vi "VP_RT_dual.vi"() -> ()   [LabVIEW 2015]
uses:
  State Enum.ctl
  Command Enum.ctl
  Controller Type.ctl
  Scan type.ctl
  EPICS Command Control.ctl
  <vilib>/Platform/TimedLoop/XDataNode/timing_clust.ctl
  <vilib>/Platform/TimedLoop/XDataNode/nitl_modes.ctl
  <vilib>/Platform/TimedLoop/XDataNode/wakeup.ctl
  Data Write Control.ctl
  <vilib>/FPGAPlugInAG/cRIO-9039/niLvFpga_Open_cRIO-9039.vi
  <vilib>/rvi/interface/common/dynamic/niFpgaDynamicAddResources.vi
  <vilib>/Utility/error.llb/Error Cluster From Error Code.vi
  <vilib>/rvi/errors/niLvFpgaAdjustHostInterfaceError.vi
  <vilib>/rvi/interface/common/niFpgaWaitOnOcc.vi
  <vilib>/FPGAPlugInAG/Dynamic/niLvFpga_Reset_Dynamic.vi
  <vilib>/FPGAPlugInAG/Dynamic/niLvFpga_Abort_Dynamic.vi
  <vilib>/FPGAPlugInAG/Dynamic/niLvFpga_Close_Dynamic.vi
  <vilib>/Platform/TimedLoop/XDataNode/XDataNode.xnode
  <vilib>/rvi/interface/nirviOpenFPGA/nirviOpenFPGA.xnode
  FPGA Bitfiles/VP_NanoPositioner_FPGA_Diagonal.lvbitx
  <vilib>/rvi/interface/nirviReadWriteControl/nirviReadWriteControl.xnode
  <vilib>/rvi/interface/nirviMethod/nirviMethod.xnode
  <vilib>/rvi/interface/nirviCloseFPGA/nirviCloseFPGA.xnode
  <vilib>/Platform/TimedLoop/XDataNode/XDNodeRunTimeDep.lvlib
  <vilib>/rvi/errors/niLvFpgaMergeErrorWithErrorCode.vi
  NiFpgaLv.dll
  <vilib>/rvi/interface/Simulation/niFpgaSimulationCallBeginRW.vi
  <vilib>/rvi/Analysis/host/Public/NI_FpgaMspHost.lvlib
  <vilib>/FPGAPlugInAG/Dynamic/niLvFpga_StopFifo_Dynamic.vi
  <vilib>/FPGAPlugInAG/Dynamic/niLvFpga_ReadFifo_Dynamic.vi
  <vilib>/NI_Real-Time Target Support.lvlib
  <vilib>/FPGAPlugInAG/Dynamic/niLvFpga_ConfigureFifo_Dynamic.vi
panel:
  in  "Tab Control":T1(tab)
  in  "Scan type":T2
  in  "Controller Type":T3
  out "Fly Scan Complete":bool
  out "XY actual":cluster{"Array":dbl[], "Array":dbl[]}(graph)
  out "XY Ref":cluster{"Array":dbl[], "Array":dbl[]}(graph)
  out "Elements Available in FIFO":u32(graph)
  out "Elements Remaining in FIFO":u32(graph)
  out "Reference and Actual positions":cluster{"t0":dbl, dbl, dbl[][]}(graph)
  in  "Timeout FPGA FIFO1":i32=40000000
  out "FIFO Timed Out":bool
  out "stop case":bool
  in  "Datalog Cases":T4(ring)=enum."Data Log 16"
  out "FIFO Timed Out?":bool
  in  "FIFO Time Period":dbl=0.01 format="%#_13g"
  out "Number of Elements":u32=1250
  out "Datalog Rate (Hz)":dbl=25000.000000000004
  out "Elements Remaining":u32
  in  "Timeout (ms)":i32=10000
  out "Actual Depth":u32=131068416
  in  "Requested Depth":u32=131068000
  out "2iddVELO:VP:X_End_nm":dbl=2000.0
  out "2iddVELO:VP:X_Start_nm":dbl=-2000.0
  out "EPICS Execute Command":bool
  out "2iddVELO:VP:Y_Start_nm":dbl=2000.0
  out "2iddVELO:VP:Y_End_nm":dbl=-2000.0
  out "2iddVELO:VP:Y_Step_Size_nm":dbl=50.0
  out "2iddVELO:VP:X_Step_Size_nm":dbl=50.0
  out "2iddVELO:VP:Trigger_Freq_Hz":dbl=1000.0
  out "2iddVELO:VP:Trig_DutyCycle_Per":dbl=99.0
  out "Iteration Duration RT Timed-Loop":i64=128
  in  "X Ramp Start (nm)":fxp<+/-,16,16>=-500.0
  in  "X Ramp End (nm)":fxp<+/-,16,16>=500.0
  in  "X Start Marker (nm)":fxp<+/-,58,25>
  in  "Y Ramp Start (nm)":fxp<+/-,16,16>=500.0
  in  "Y Ramp End (nm)":fxp<+/-,16,16>=-500.0
  in  "Y Step Size (nm)":fxp<+/-,16,16>=50.0
  in  "Y Start Marker (nm)":fxp<+/-,58,25>
  out "Fly Scan Running":bool
  out "Continue Run":bool
  out "X Ramp Period (usec)":fxp<+,24,24>=60000.0
  out "Y Ramp Period (usec)":fxp<+,24,24>=60000.0
  out "# of Hor Lines":fxp<+/-,34,18>=181.0 format="%.22g"
  in  "X Step Size (nm)":fxp<+/-,16,16>=50.0
  out "# of Points per Line":fxp<+/-,33,17>=180.0
  out "# Total Trigger Points":fxp<+/-,64,34>=32580.0
  out "sec per line":dbl=0.06
  out "line per sec (Hz)":dbl=16.666666666666668
  out "X Ramp Period DBL (usec)":dbl=60000.0 format="%#_6f"
  out "Total Scan Time (sec)":dbl=10.86
  in  "Controller Time Period (uSec)":u32=40
  in  "Controller Output Time Period (uSec)":u32=40
  in  "X Reference Time Period (uSec)":u32=40
  in  "Plant Output Time Period (uSec)":u32=40
  in  "Stop System (Careful!!)":bool
  in  "Datalog Time Period (uSec)":u32=40
  in  "Analog Input Time Period (uSec)":u32=40
  in  "Detector Trigger Time Period (uSec)":u32=40
  in  "Trigger Generation Time Period (uSec)":u32=40
  in  "Y Reference Time Period (uSec)":u32=40
  in  "Z Reference Time Period (uSec)":u32=40
  in  "Data Trigger Time Period (uSec)":u32=40
  in  "Reset All":bool
  in  "System Loop Type":enum16{"Open Loop", "Closed Loop"}(ring)
  in  "Base name":string="base_name"
  out "Trigger for Data":fxp<+/-,58,25>=1.0
  out "Data":fxp<+/-,58,25>[](array[numeric])
  out "Number of Data Strings":i32=5
  out "Mod6/DIO3":bool
  out "Mod5/DIO3":bool
  out "Mod4/DIO3":bool
  in  "Sample Z Stage Resolution (nm)":fxp<+,33,3>=0.5
  in  "Sample Y Stage Resolution (nm)":fxp<+,33,3>=0.5
  in  "Sample X Stage Resolution (nm)":fxp<+,33,3>=0.5
  in  "Optics Z Stage Resolution (nm)":fxp<+,33,3>=0.5
  in  "Optics Y Stage Resolution (nm)":fxp<+,33,3>=0.5
  in  "Optics X Stage Resolution (nm)":fxp<+,33,3>=0.5
  in  "Sample Z Reset":bool
  in  "Sample Y Reset":bool
  in  "Sample X Reset":bool
  out "Mod6/DIO2":bool
  out "Mod6/DIO1":bool
  out "Mod6/DIO0":bool=TRUE
  out "Mod5/DIO2":bool
  out "Mod5/DIO1":bool=TRUE
  out "Mod5/DIO0":bool
  out "Mod4/DIO2":bool=TRUE
  out "Mod4/DIO1":bool
  out "Mod4/DIO0":bool=TRUE
  in  "Optics Z Reset":bool
  in  "Optics Y Reset":bool
  in  "Optics X Reset":bool
  in  "Detector Trigger Lower Limit (V)":fxp<+/-,20,5>
  in  "Detector Trigger Upper Limit (V)":fxp<+/-,20,5>=5.0
  out "Detector Trigger (V)":fxp<+/-,20,5>
  out "Detector Trigger In Range?":bool=TRUE
  in  "Trigger High Period (usec)":fxp<+/-,64,45>=1250.0
  in  "Trigger Low Period (usec)":fxp<+/-,64,45>=1250.0
  in  "Trigger High Level (V)":fxp<+/-,20,5>=5.0
  in  "Trigger Low Level (V)":fxp<+/-,20,5>
  in  "Trigger Wave Generator":T5(ring)=enum."Square Wave 1"
  in  "DT Reference Amplitude (V)":fxp<+/-,40,17>=5.0
  in  "DT Reference DC Offset (V)":fxp<+/-,16,16>
  out "DT Frequency (periods/tick)":fxp<+,32,0>=7.500010542571545e-05
  out "DT Phase Offset (periods)":fxp<+,32,0>
  in  "DT Reset":bool
  out "DT Duty Cycle (periods)":fxp<+,32,0>=0.8799999998882413
  in  "DT phase offset (deg)":dbl format="%#.6g"
  in  "DT Frequency (Hz)":dbl=200.0 format="%#_6p"
  in  "DT duty cycle (%)":dbl=88.0 min=0.0 max=100.0 step=1.0
  in  "Z White Noise Seed":u32=4
  in  "Z White Noise Amplitude":u16=32767
  in  "Y White Noise Seed":u32=4
  in  "Y White Noise Amplitude":u16=32767
  in  "Z Reference Reset":bool
  in  "Y Reference Reset":bool
  in  "X Reference Reset":bool
  in  "Z Reference Wave Selection":T6(ring)=enum."Sine Wave"
  in  "X Reference Wave Selection":T7(ring)=enum."Custom Up Down Ramp"
  in  "Y Reference Wave Selection":T8(ring)=enum."Custom Ramp Wave"
  out "Z phase offset (periods)":fxp<+,32,0>
  out "Z frequency (periods/tick)":fxp<+,32,0>=1.25030055642128e-07 format="%.32g"
  in  "Z phase offset (deg)":dbl format="%#.6g"
  in  "Z frequency (Hz)":dbl=5.0 format="%#_6p"
  out "Y phase offset (periods)":fxp<+,32,0>
  out "Y frequency (periods/tick)":fxp<+,32,0>=5.005858838558197e-08 format="%.32g"
  in  "Y phase offset (deg)":dbl format="%#.6g"
  in  "Y frequency (Hz)":dbl=2.0 format="%#_6p"
  out "Z Stage Reference (nm)":fxp<+/-,58,25>
  out "Y Stage Reference (nm)":fxp<+/-,58,25>
  out "X Stage Reference (nm)":fxp<+/-,58,25>
  in  "X White Noise Seed":u32=4
  in  "X White Noise Amplitude":u16=32767
  in  "Z Reference DC Offset (nm)":fxp<+/-,15,15>
  in  "Y Reference DC Offset (nm)":fxp<+/-,16,16>
  in  "X Reference DC Offset (nm)":fxp<+/-,16,16>
  in  "Z Reference Amplitude (nm)":fxp<+/-,40,17>
  in  "Y Reference Amplitude (nm)":fxp<+/-,40,17>=100.0
  in  "X Reference Amplitude (nm)":fxp<+/-,40,17>=100.0
  out "X phase offset (periods)":fxp<+,32,0>
  out "X frequency (periods/tick)":fxp<+,32,0>=1.25030055642128e-07 format="%.32g"
  in  "X phase offset (deg)":dbl format="%#.6g"
  in  "X frequency (Hz)":dbl=5.0 format="%#_6p"
  in  "Scaling mV to V":fxp<+,33,10>=0.001000046730041504
  out "Heartbeat":bool=TRUE
  in  "System command":T9
  in  "Execute":bool
  out "Last Command Executed":T9
  in  "Optics and or Sample Stage":T10(ring)
  out "Remote Mode":bool
  in  "Local_Lock":bool
  out "Snake Scan Reference FPGA or EPICS":enum16{"FPGA Snake Scan", "EPICS Snake Scan"}(ring)
  out "Output filename":string
  out "Output path":path
  out "FPGA state":T11(ring)
  in  "cRIO data dir":string="/home/lvuser/natinst/data"
  out "RT Main Loop State":T12
  out "cRIO path":path
  out "Trigger Frequency (Hz)":dbl
  out "Trigger Duty Cycle (%)":dbl
  out "EPICS Scan Type":T2
  out "EPICS Controller Type":T3
  out "EPICS cRIO Command":T13
  out "Scan loop dt":i64
  in  "Z-Stage Scaling Direction":fxp<+/-,3,3>=-1.0
  in  "Y-Stage Scaling Direction":fxp<+/-,3,3>=-1.0
  in  "Mod 3 AI2 V to nm Scaling":fxp<+,47,18>=1000.0
  in  "Mod 3 AI1 V to nm Scaling":fxp<+,47,18>=1000.0
  in  "Mod 3 AI0 V to nm Scaling":fxp<+,47,18>=1000.0
  out "PI Z-Stage Input (V)":fxp<+/-,20,5>=-0.000732421875
  out "PI Y-Stage Input (V)":fxp<+/-,20,5>=0.005584716796875
  out "PI X-Stage Input (V)":fxp<+/-,20,5>=-0.00311279296875
  in  "Z-Stage nm to V Scaling":fxp<+/-,32,12>=0.0005397796630859375
  in  "Y-Stage nm to V Scaling":fxp<+/-,32,12>=0.0014200210571289062
  in  "X-Stage Scaling Direction":fxp<+/-,3,3>=-1.0
  in  "X-Stage nm to V Scaling":fxp<+/-,32,12>=0.0005359649658203125
  in  "Controller Output Lower Limit":fxp<+/-,20,5>=-5.0
  in  "Controller Output Upper Limit":fxp<+/-,20,5>=5.0
  in  "FPGA Wait Timer (ms)":u16=50
  in  "Pre-Scan pause (ms)":u32=250
  in  "Readback Loop time between iterations (ms)":u32=10
  out "Measured Datalog Time Period (Ticks)":u32=1600
  out "Measured Datalog Loop Rate (secs)":dbl=3.9999999999999996e-05
  out "Measured Datalog Loop Rate (kHz)":dbl=25.000000000000004
  out "Measured Counter Loop Rate (secs)":dbl
  out "Measured Counter Loop Rate (MHz)":dbl=inf
  out "Measured X Reference Loop Rate (secs)":dbl=3.9999999999999996e-05
  out "Measured X Reference Loop Rate (kHz)":dbl=25.000000000000004
  out "Measured X Reference Time Period (Ticks)":u32=1600
  out "Measured Controller Loop Rate (kHz)":dbl=25.000000000000004
  out "Measured Controller Output Loop Rate (secs)":dbl=3.9999999999999996e-05
  out "Measured Controller Output Loop Rate (kHz)":dbl=25.000000000000004
  out "Measured Plant Output Loop Rate (secs)":dbl=3.9999999999999996e-05
  out "Measured Plant Output Loop Rate (kHz)":dbl=25.000000000000004
  out "Measured Controller Loop Rate (secs)":dbl=3.9999999999999996e-05
  out "Measured Controller Time Period (Ticks)":u32=1600
  out "Datalog Time Period (sec)":dbl=3.9999999999999996e-05
  out "Measured Controller Output Time Period (Ticks)":u32=1600
  out "Measured Plant Output Time Period (Ticks)":u32=1600
  out "Measured Counter Time Period (Ticks)":u32
  out "32 bit Count Optics X":i32
  out "32 bit Count Optics  Y":i32
  out "32 bit Count Optics  Z":i32
  out "32 bit Count Sample X":i32
  out "32 bit Count Sample  Y":i32=2
  out "32 bit Count Sample  Z":i32=-4
  out "Optics X Stage Displacement (nm)":fxp<+/-,58,25>=-1.0
  out "Optics Y Stage Displacement (nm)":fxp<+/-,58,25>
  out "Optics Z Stage Displacement (nm)":fxp<+/-,58,25>
  out "Sample X Stage Displacement (nm)":fxp<+/-,58,25>=-0.5
  out "Sample Y Stage Displacement (nm)":fxp<+/-,58,25>=1.5
  out "Sample Z Stage Displacement (nm)":fxp<+/-,58,25>=-1.0
  out "Measured Analog Input Time Period (Ticks)":u32=1600
  out "Measured Analog Input Loop Rate (secs)":dbl=3.9999999999999996e-05
  out "Measured Analog Input Loop Rate (kHz)":dbl=25.000000000000004
  out "Measured Detector Trigger Time Period (Ticks)":u32=1600
  out "Measured Trigger Gen Time Period (Ticks)":u32=1600
  out "Measured Y Reference Time Period (Ticks)":u32=1600
  out "Measured Z Reference Time Period (Ticks)":u32=1600
  out "Measured Y Reference Loop Rate (secs)":dbl=3.9999999999999996e-05
  out "Measured Y Reference Loop Rate (kHz)":dbl=25.000000000000004
  out "Measured Z Reference Loop Rate (secs)":dbl=3.9999999999999996e-05
  out "Measured Z Reference Loop Rate (kHz)":dbl=25.000000000000004
  out "Measured Data Trigger Time Period (Ticks)":u32=1600
  out "X-Stage Input In Range?":bool=TRUE
  out "Y-Stage Input In Range?":bool=TRUE
  out "Z-Stage Input In Range?":bool=TRUE
  in  "file path soscoeff_xx1 Hinf":path=path "/home/lvuser/natinst/controllers/Kxx_1_Gxx_matched_dow_16ord_mVpnm_cd8a3_AvTio9_X5nm_500pm_all_40us_soscof_xx1.mat"
  in  "file path sos gain SF Controller_xx1 Hinf":path=path "/home/lvuser/natinst/controllers/Kxx_1_Gxx_matched_dow_16ord_mVpnm_cd8a3_AvTio9_X5nm_500pm_all_40us_soscof_xx2.mat"
  in  "file path soscoeff_yy1 Hinf":path=path "/home/lvuser/natinst/controllers/Kyy_trial_1_Gyy_matched_dow_8ord_mVpnm_cd8a3_AvTio9_Y5nm_500pm_all_40us_soscof_yy1.mat"
  in  "file path sos gain SF Controller_yy1 Hinf":path=path "/home/lvuser/natinst/controllers/Kyy_trial_1_Gyy_matched_dow_8ord_mVpnm_cd8a3_AvTio9_Y5nm_500pm_all_40us_soscof_yy2.mat"
  in  "file path soscoeff_zz1 Hinf":path=path "/home/lvuser/natinst/controllers/Kzz_1_Gzz_matched_dow_29ord_mVpnm_cd8a3_AvTio9_Z5nm_500pm_all_40us_soscof_zz1.mat"
  in  "file path sos gain SF Controller_zz1 Hinf":path=path "/home/lvuser/natinst/controllers/Kzz_1_Gzz_matched_dow_29ord_mVpnm_cd8a3_AvTio9_Z5nm_500pm_all_40us_soscof_zz2.mat"
  in  "file path soscoeff_xx1 PID":path=path "/home/lvuser/natinst/controllers/Kxx_pid_2_Gxx_tustin_2ord_mVpnm_cd8a3_soscof_xx1.mat"
  in  "file path sos gain SF Controller_xx1 PID":path=path "/home/lvuser/natinst/controllers/Kxx_pid_2_Gxx_tustin_2ord_mVpnm_cd8a3_soscof_xx2.mat"
  in  "file path soscoeff_yy1 PID":path=path "/home/lvuser/natinst/controllers/Kyy_pid_4_Gyy_tustin_2ord_mVpnm_cd8a3_soscof_yy1.mat"
  in  "file path sos gain SF Controller_yy1 PID":path=path "/home/lvuser/natinst/controllers/Kyy_pid_4_Gyy_tustin_2ord_mVpnm_cd8a3_soscof_yy2.mat"
  in  "file path soscoeff_zz1 PID":path=path "/home/lvuser/natinst/controllers/Kzz_pid_2_Gzz_tustin_2ord_mVpnm_cd8a3_soscof_zz1.mat"
  in  "file path sos gain SF Controller_zz1 PID":path=path "/home/lvuser/natinst/controllers/Kzz_pid_2_Gzz_tustin_2ord_mVpnm_cd8a3_soscof_zz2.mat"
  out "-a01(2) xx1c":fxp<+/-,64,9>[](array[numeric])=[0.637785025840232, 0.9924182654286198, 1.8461027816316544, 0.8635404845716299, 1.0670555456779864, 1.6350703383821101, 1.6323955588345012, 1.1102241390539636, 0.0, 0.0, 0.0, 0.0, 0.0, 0.0, 0.0, 0.0, 0.0, 0.0, 0.0, 0.0]
  out "-a02(2) xx1c":fxp<+/-,64,9>[](array[numeric])=[-0.999855815746439, -0.9676991072632725, -0.9642268720534838, -0.9446498323360957, -0.9442808087139987, -0.7547983908829242, -0.6690016013017409, -0.11027986125857198, 0.0, 0.0, 0.0, 0.0, 0.0, 0.0, 0.0, 0.0, 0.0, 0.0, 0.0, 0.0]
  out "b01(2) xx1c":fxp<+/-,64,9>[](array[numeric])=[-0.6378105164532328, -1.0062332697665268, -1.8762916543815855, -0.8616288879491845, -1.0856571140792324, -1.6862585929720944, -1.743591709663851, -0.6129835805090948, 0.0, 0.0, 0.0, 0.0, 0.0, 0.0, 0.0, 0.0, 0.0, 0.0, 0.0, 0.0]
  out "b02(2) xx1c":fxp<+/-,64,9>[](array[numeric])=[0.9999102047610771, 0.9971375605901365, 0.9926840301018772, 0.9509648854364836, 0.9563369558920378, 0.7818900462139817, 0.7642575436257291, 3.0531133177191805e-16, 0.0, 0.0, 0.0, 0.0, 0.0, 0.0, 0.0, 0.0, 0.0, 0.0, 0.0, 0.0]
  out "sos gain SF Controller xx1c":fxp<+/-,42,9>=-0.1625035791657865
  out "-a01(2) yy1c":fxp<+/-,64,9>[](array[numeric])=[1.8740229377643998, 1.3096977339382483, 1.7453886241944765, 0.2668895009727739, 0.0, 0.0, 0.0, 0.0, 0.0, 0.0, 0.0, 0.0, 0.0, 0.0, 0.0, 0.0, 0.0, 0.0, 0.0, 0.0]
  out "-a02(2) yy1c":fxp<+/-,64,9>[](array[numeric])=[-0.9732703278433918, -0.5194903821190732, -0.7453924481836136, -2.7755575615628914e-17, 0.0, 0.0, 0.0, 0.0, 0.0, 0.0, 0.0, 0.0, 0.0, 0.0, 0.0, 0.0, 0.0, 0.0, 0.0, 0.0]
  out "b01(2) yy1c":fxp<+/-,64,9>[](array[numeric])=[-1.8979173162254057, -1.8463149313261074, -1.7151162246453355, -0.006444279582847878, 0.0, 0.0, 0.0, 0.0, 0.0, 0.0, 0.0, 0.0, 0.0, 0.0, 0.0, 0.0, 0.0, 0.0, 0.0, 0.0]
  out "b02(2) yy1c":fxp<+/-,64,9>[](array[numeric])=[0.9969084979865663, 0.9421233904433339, 0.7362048104846675, 0.0, 0.0, 0.0, 0.0, 0.0, 0.0, 0.0, 0.0, 0.0, 0.0, 0.0, 0.0, 0.0, 0.0, 0.0, 0.0, 0.0]
  out "sos gain SF Controller yy1c":fxp<+/-,42,9>=-1.480983349494636
  out "-a01(2) zz1c":fxp<+/-,64,9>[](array[numeric])=[0.6242394224317618, 1.8967038692417004, 0.6659160318030806, 1.7792660019034106, 1.6870099721477447, 0.6417945190222861, 1.4838029149808185, 1.8456549628851837, 1.2189509782386598, 0.9933314517253298, 1.0158915520299678, 0.8863484387433826, 0.026837806879254994, 1.8269783715122585, 0.22448441435364225, 0.0, 0.0, 0.0, 0.0, 0.0]
  out "-a02(2) zz1c":fxp<+/-,64,9>[](array[numeric])=[-0.9983298461163967, -0.9972287452752734, -0.995744457243837, -0.9947210838396919, -0.9925914602095722, -0.9920974045271405, -0.9881915357970101, -0.9800069383591395, -0.9760641145386646, -0.9508624135515895, -0.9242774595356998, -0.655945641403593, -0.008661844724279444, -0.8269827070369743, 0.0, 0.0, 0.0, 0.0, 0.0, 0.0]
  out "b01(2) zz1c":fxp<+/-,64,9>[](array[numeric])=[-0.6245671059510156, -1.897930093390194, -0.6670970070931089, -1.7670265604573054, -1.6833314913922348, -0.6327437892303018, -1.5025901530730128, -1.8636454269915796, -1.1210694827766767, -0.9982206064398196, -1.0326369335418408, -1.1342635673267367, -1.6852506306166828, -0.9843740162364313, -1.7208456881689926e-15, 0.0, 0.0, 0.0, 0.0, 0.0]
  out "b02(2) zz1c":fxp<+/-,64,9>[](array[numeric])=[0.9973135069419645, 0.9951302056171929, 0.9993435624612031, 0.9919371251860779, 0.994931751453586, 0.9881092761723503, 0.9884874399279107, 0.9977145546300196, 0.9725302934743221, 0.9855561672767964, 0.9893454712398023, 0.846212786518208, 0.7855598927779743, 0.0978075435519738, 0.0, 0.0, 0.0, 0.0, 0.0, 0.0]
  out "sos gain SF Controller zz1c":fxp<+/-,42,9>=-0.1988595259608701
  out "error out (Sig Gen)":errorcluster
  out "FPGA error monitor":errorcluster
  out "FPGA end run error":errorcluster
  out "Timed Loop (end error)":errorcluster
  out "error out (Sig Gen) 2":errorcluster
  out "error out (Sig Gen) 3":errorcluster
  out "error out (Sig Gen) 4":errorcluster
  out "Main Loop error":errorcluster
  out "Main Loop Iterations":i32
  out "RT error":errorcluster
  out "Command Loop Error":errorcluster
  out "Readback error":errorcluster
  out "FPGA wait error":errorcluster
  out "Coeff file import error":errorcluster
  out "Readback loop Iterations":i32
  out "Command Loop Iterations":i32
  out "Heartbeat Loop Iterations":i32
  out "EPICS command error":errorcluster
  out "Reduced Array of States":T12[](array[typedef])
  out "2iddVELO:VP:Scan_Type":string
  out "2iddVELO:VP:Controller_Type":string
  out "2iddVELO:VP:cRIO_Command":string
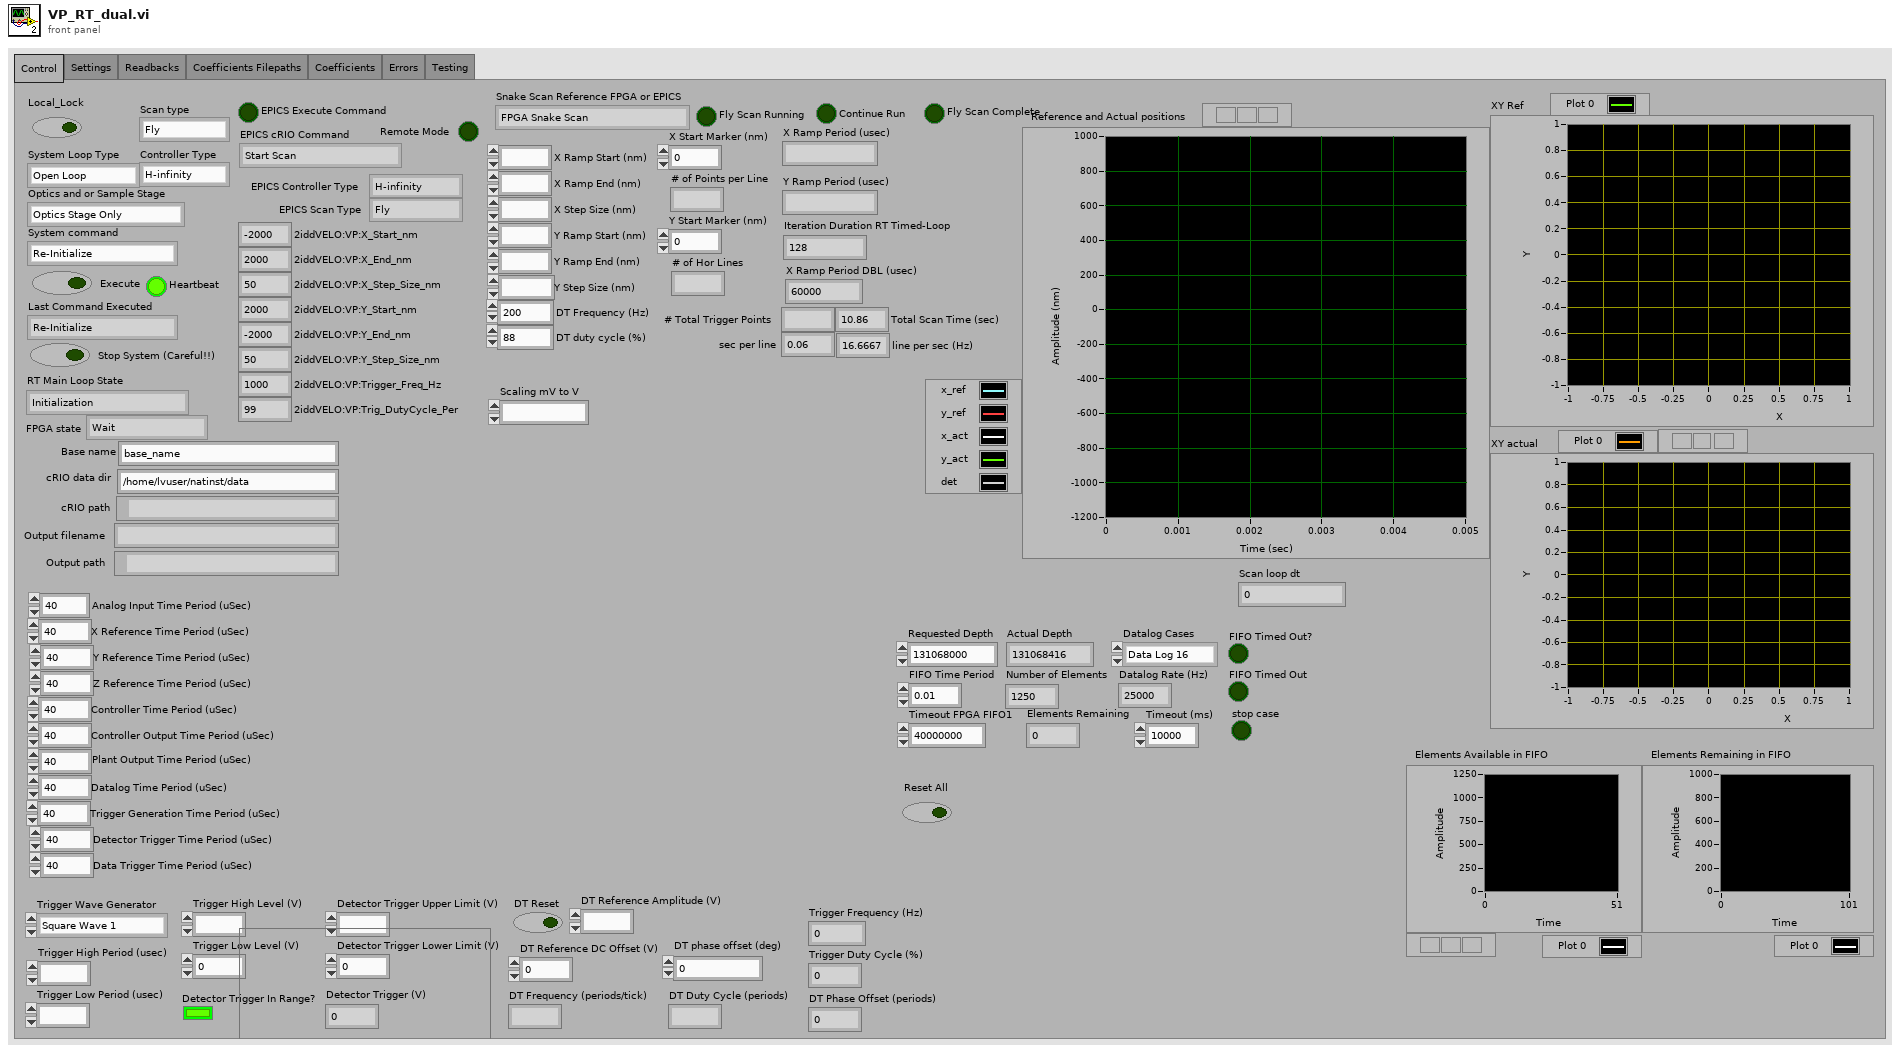
[diagram p1: front panel]
types:
  T1 = enum32{"Control", "Settings", "Readbacks", "Coefficients Filepaths", "Coefficients", "Errors", "Testing"}
  T2 = typedef "Scan type.ctl" = enum16{"Fly", "Step"}
  T3 = typedef "Controller Type.ctl" = enum16{"H-infinity", "PID"}
  T4 = enum16{"Data Log 1", "Data Log 2", "Data Log 3", "Data Log 4", "Data Log 5", "Data Log 6", "Data Log 7", "Data Log 8", "Data Log 9", "Data Log 10", "Data Log 11", "Data Log 12", "Data Log 13", "Data Log 14", "Data Log 15", "Data Log 16"}
  T5 = enum16{"Custom Square Wave ", "Square Wave 1", "Square Wave 2"}
  T6 = enum16{"Constant", "Sine Wave", "Sawtooth Wave", "Square Wave", "Filtered White Noise"}
  T7 = enum16{"Constant", "Sine Wave", "Custom Up Down Ramp", "Filtered White Noise"}
  T8 = enum16{"Constant", "Sine Wave", "Custom Ramp Wave", "Filtered White Noise"}
  T9 = typedef "Command Enum.ctl" = enum16{"Re-Initialize ", "Update Scan Settings", "Scan", "Stop Scan", "Restart FPGA", "Stop System"}
  T10 = enum16{"Optics Stage Only", "Optics and Sample Stage"}
  T11 = enum16{"Wait", "Start Run", "Run", "End Run", "Shutdown"}
  T12 = typedef "State Enum.ctl" = enum16{"Initialization", "Import Controller coeffs", "Update Controller Info", "Wait", "Update Reference Info", "Update Detector Trigger Info", "Update Datalog Info", "Check FPGA Status", "Pre-Scan", "Start Scan", "Scanning", "End Scan", "Restart FPGA", "Stop FPGA"}
  T13 = typedef "EPICS Command Control.ctl" = enum16{"Start Scan", "Stop Scan", "Reload Controller"}
  T14 = typedef "XDNodeRunTimeDep.lvlib/timing_clust.ctl" = cluster{"Expected End [f-1]":u64, "Actual End [f-1]":u64, "Finished Late? [f-1]":bool, "Expected End [i-1]":u64, "Actual End [i-1]":u64, "Finished Late? [i-1]":bool, "Expected Start [i]":u64, "Actual Start [i]":u64, "Expected Start [f]":u64, "Actual Start [f]":u64, "Source Name":string, "Structure Name":string, "Period":i64, "Deadline":i64, "Offset":i64, "Start":i64, "Priority":i32, "Timeout":i32, "Mode":T15, "Wakeup Reason":T16, "Error":errorcluster, "Source Type":string, "Secondary Source Type":string, "Global End Time":u64, "Global Start Time":u64, "Frame Duration":u64, "Iteration Duration":u64, "Assigned CPU":i32, "I/O Scan Engine Mode":u32}
  T15 = typedef "XDNodeRunTimeDep.lvlib/nitl_modes.ctl" = enum32{"No Change", "Process missed periods, maintain original phase", "Discard missed periods, maintain original phase", "Process missed periods, ignore original phase", "Discard missed periods, ignore original phase"}
  T16 = typedef "XDNodeRunTimeDep.lvlib/wakeup.ctl" = enum32{"Normal", "Aborted", "Asynchronous wakeup", "Timing source error", "Timed loop error", "Timeout"}
  T17 = typedef "Data Write Control.ctl" = enum16{"Initialize", "Read", "Write", "Close"}
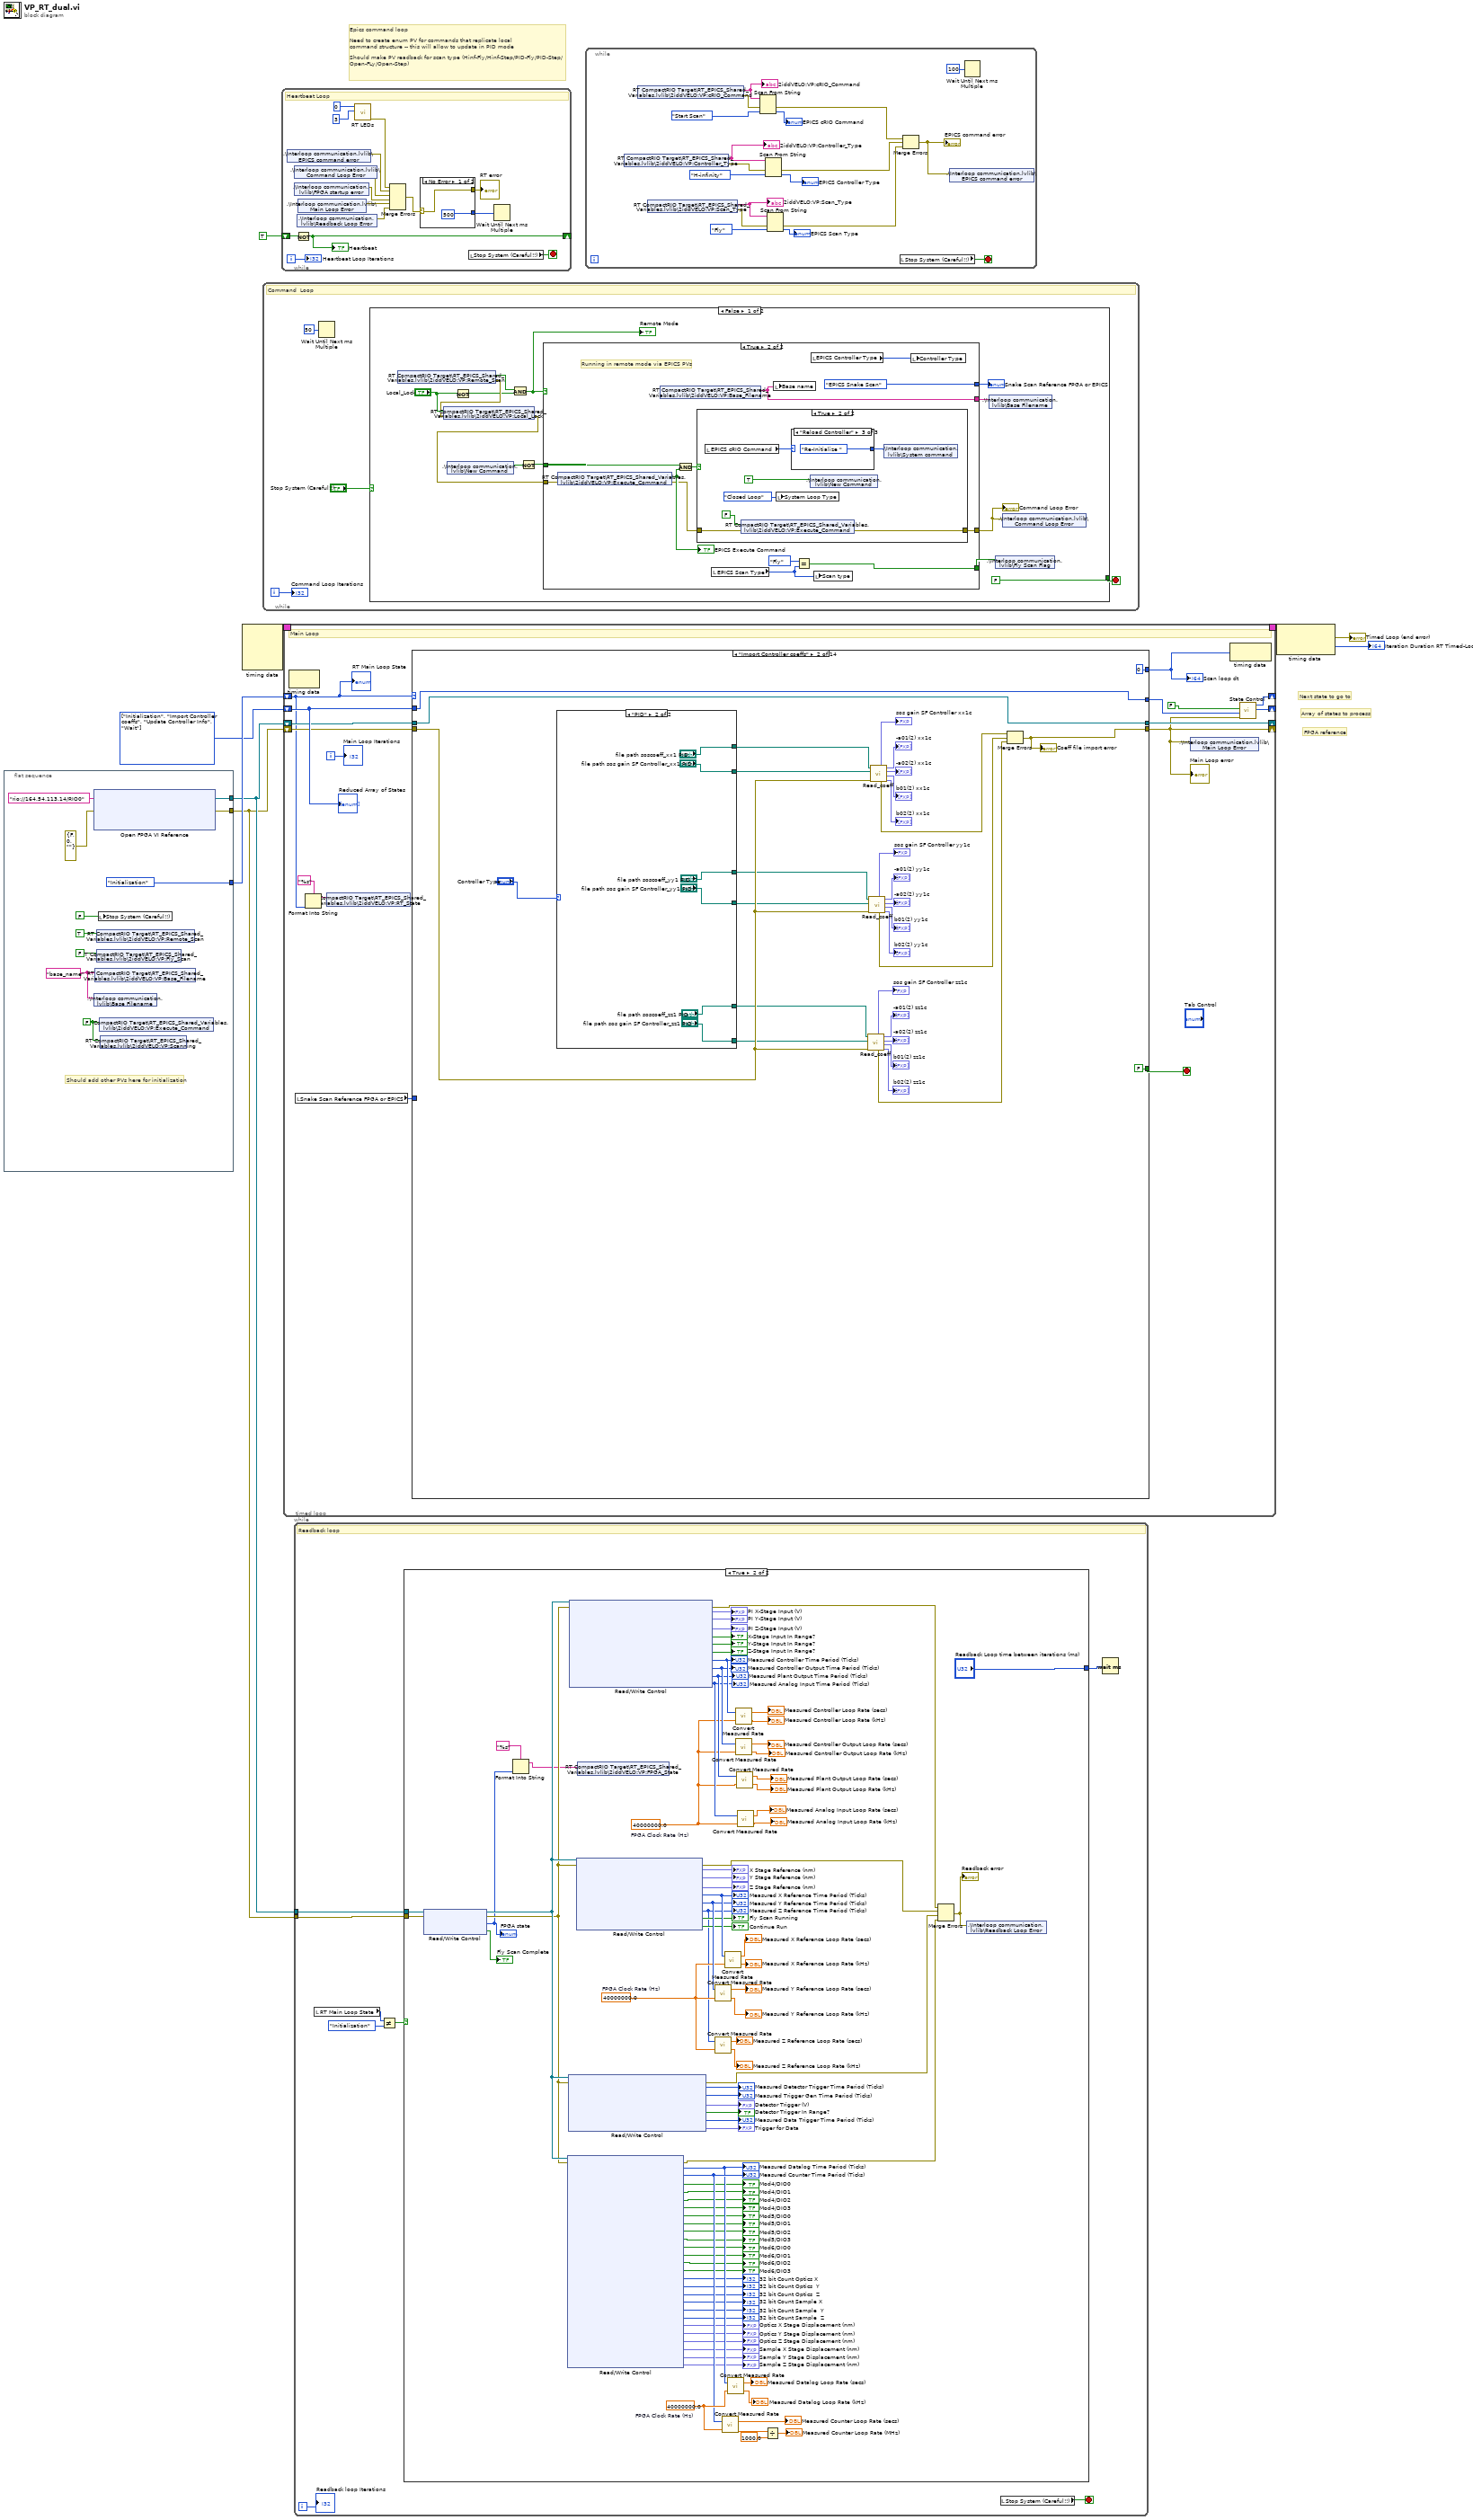
[diagram p0: block diagram]
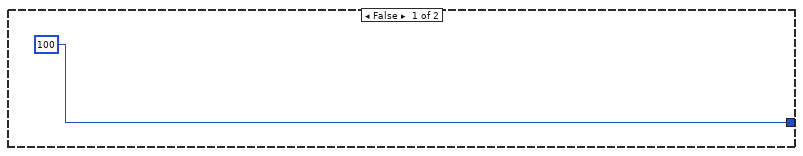
[diagram p2: hidden frame]
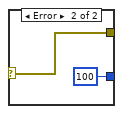
[diagram p3: hidden frame]
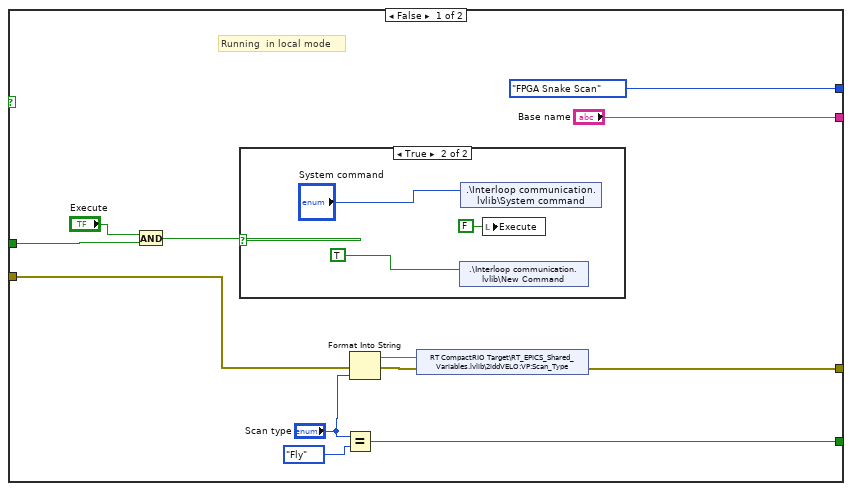
[diagram p4: hidden frame]
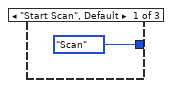
[diagram p7: hidden frame]
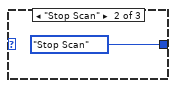
[diagram p8: hidden frame]
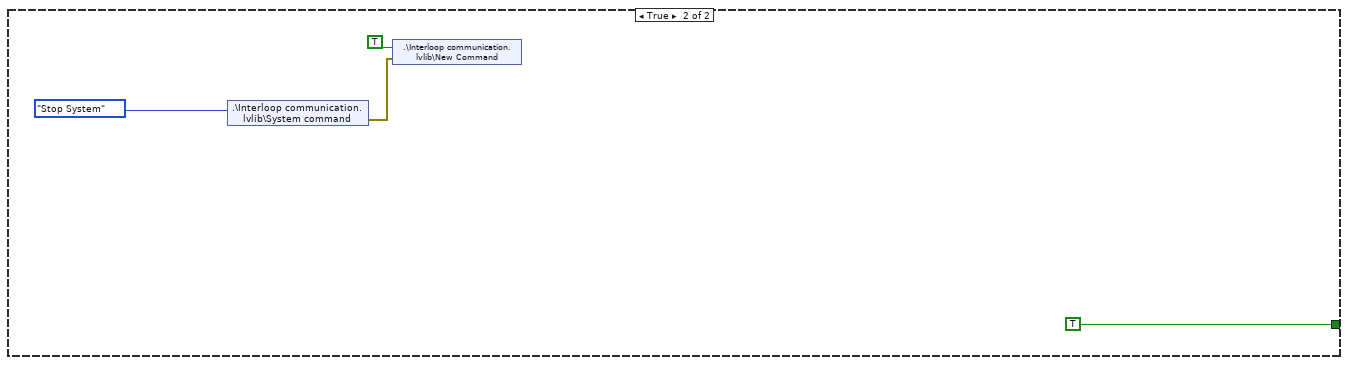
[diagram p9: hidden frame]
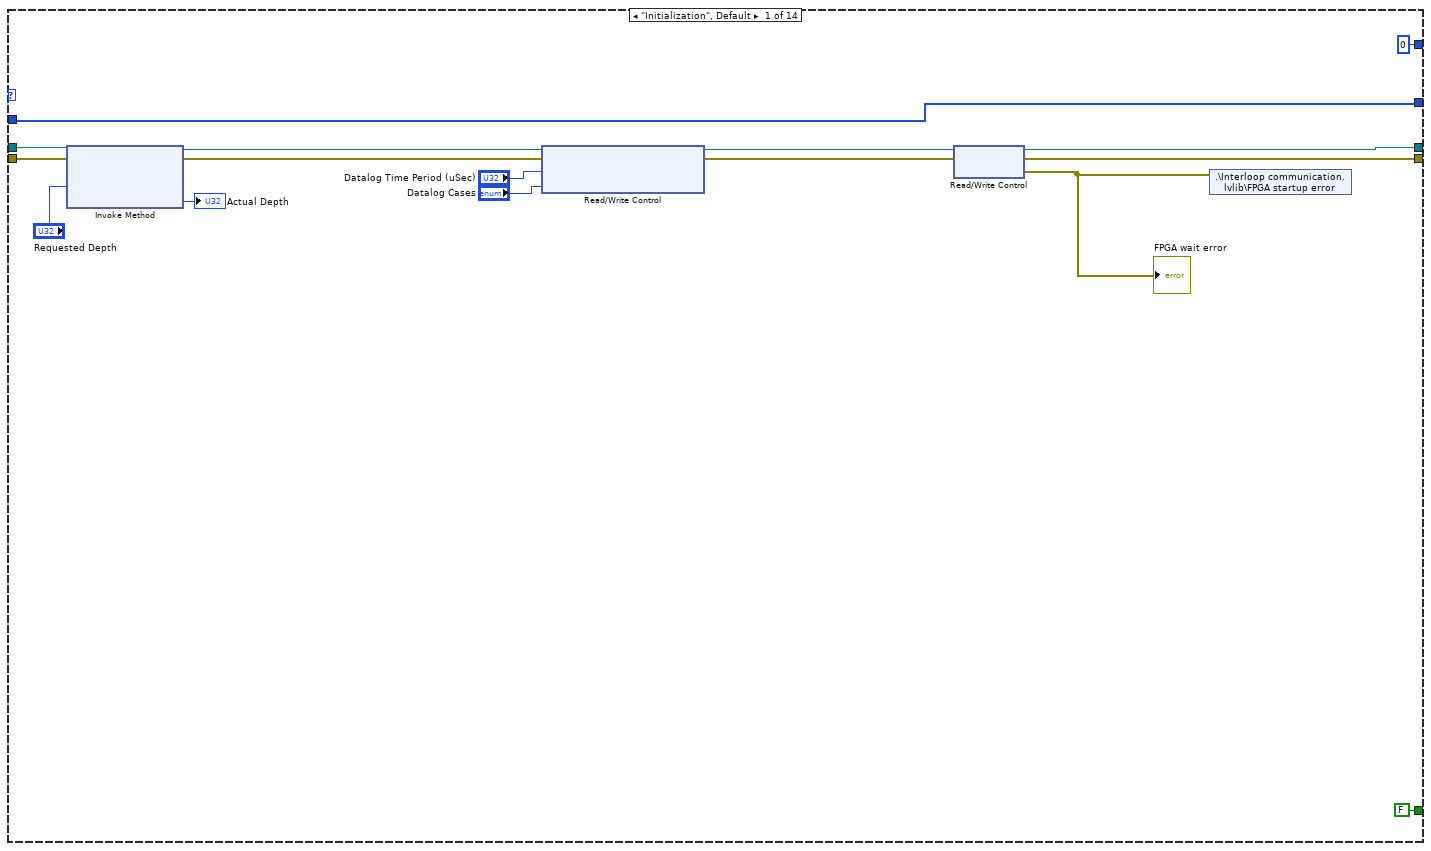
[diagram p10: hidden frame]
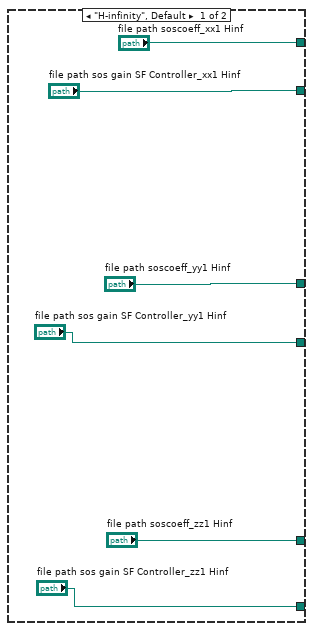
[diagram p11: hidden frame]
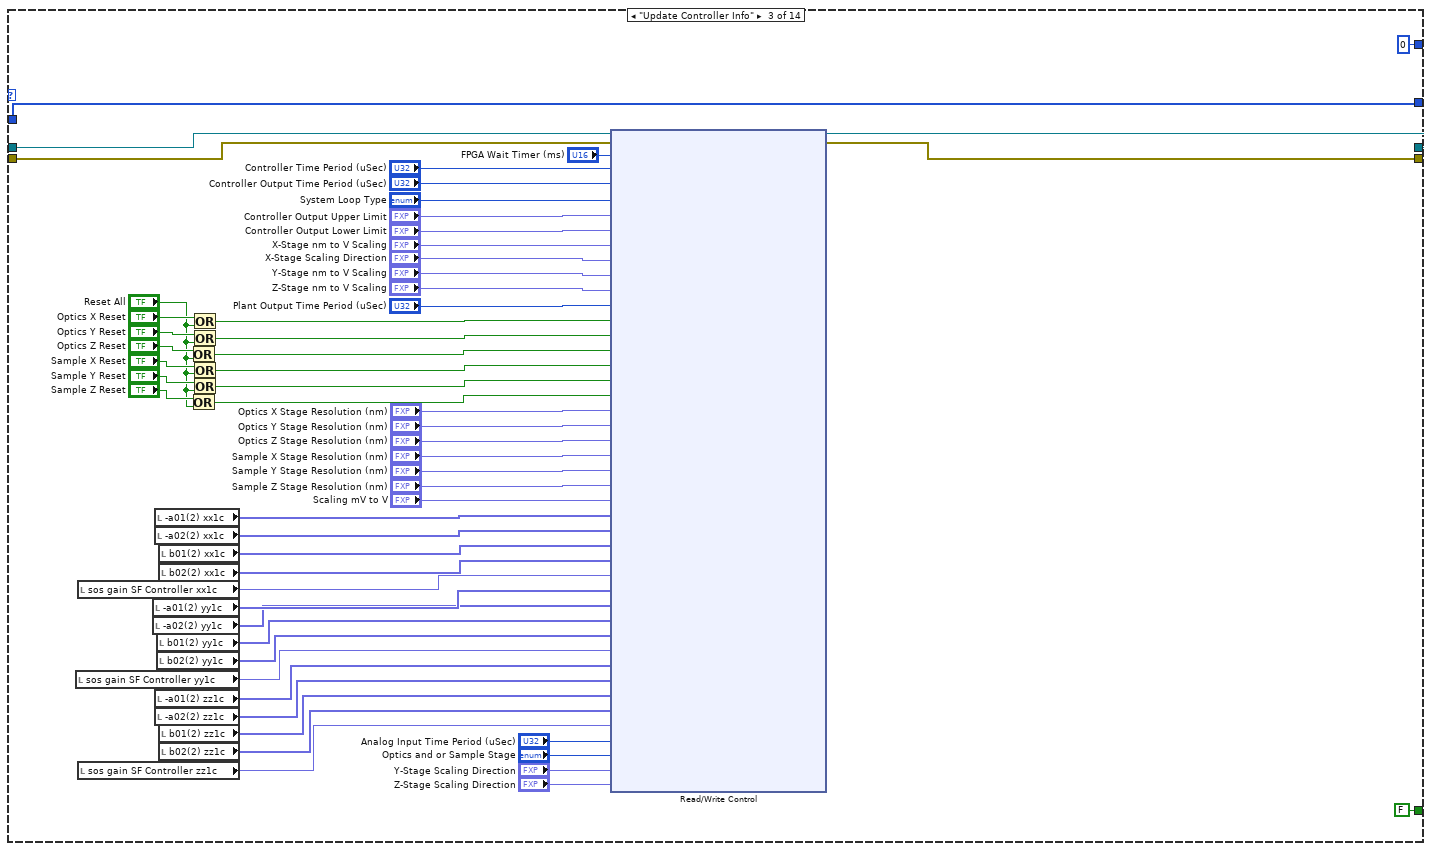
[diagram p12: hidden frame]
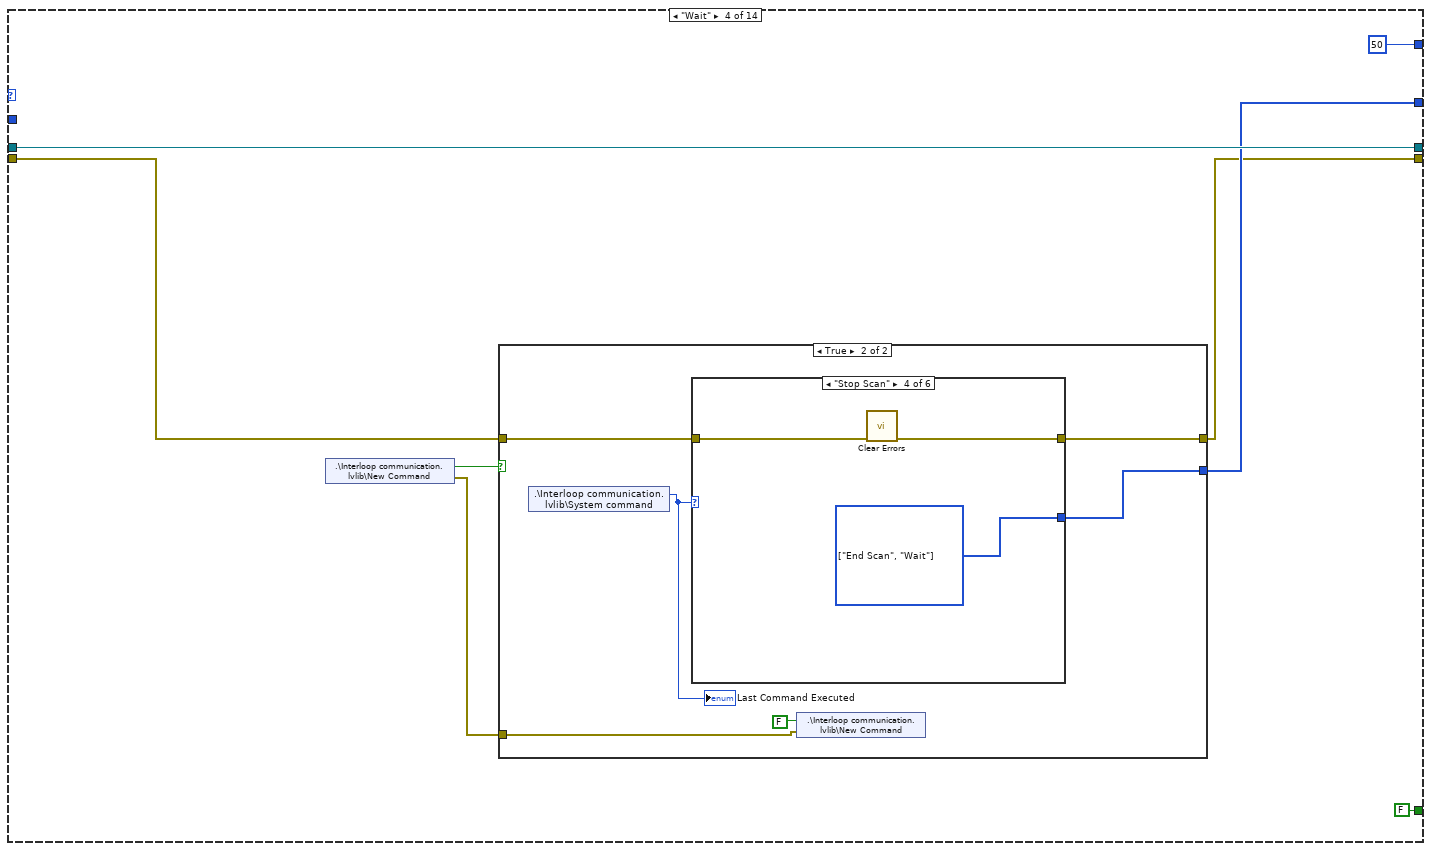
[diagram p13: hidden frame]
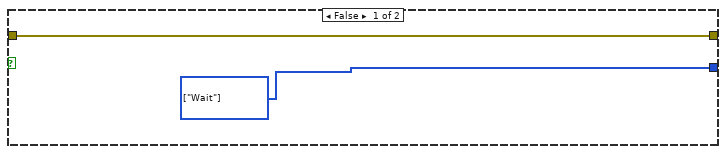
[diagram p14: hidden frame]
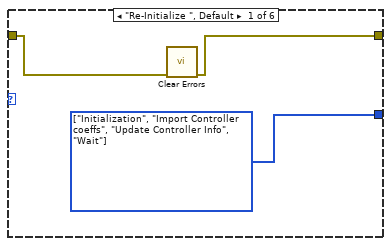
[diagram p15: hidden frame]
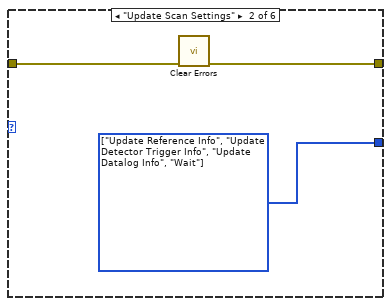
[diagram p16: hidden frame]
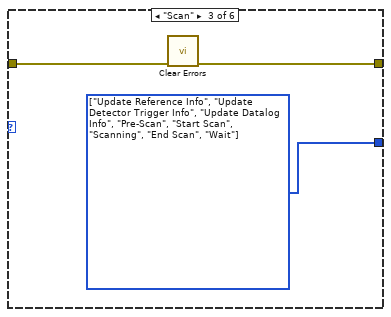
[diagram p17: hidden frame]
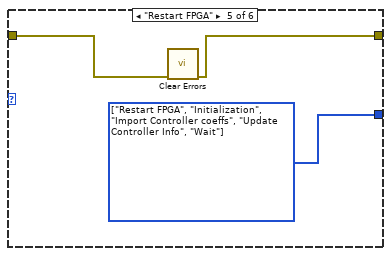
[diagram p18: hidden frame]
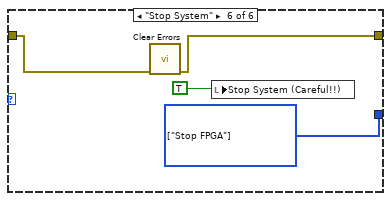
[diagram p19: hidden frame]
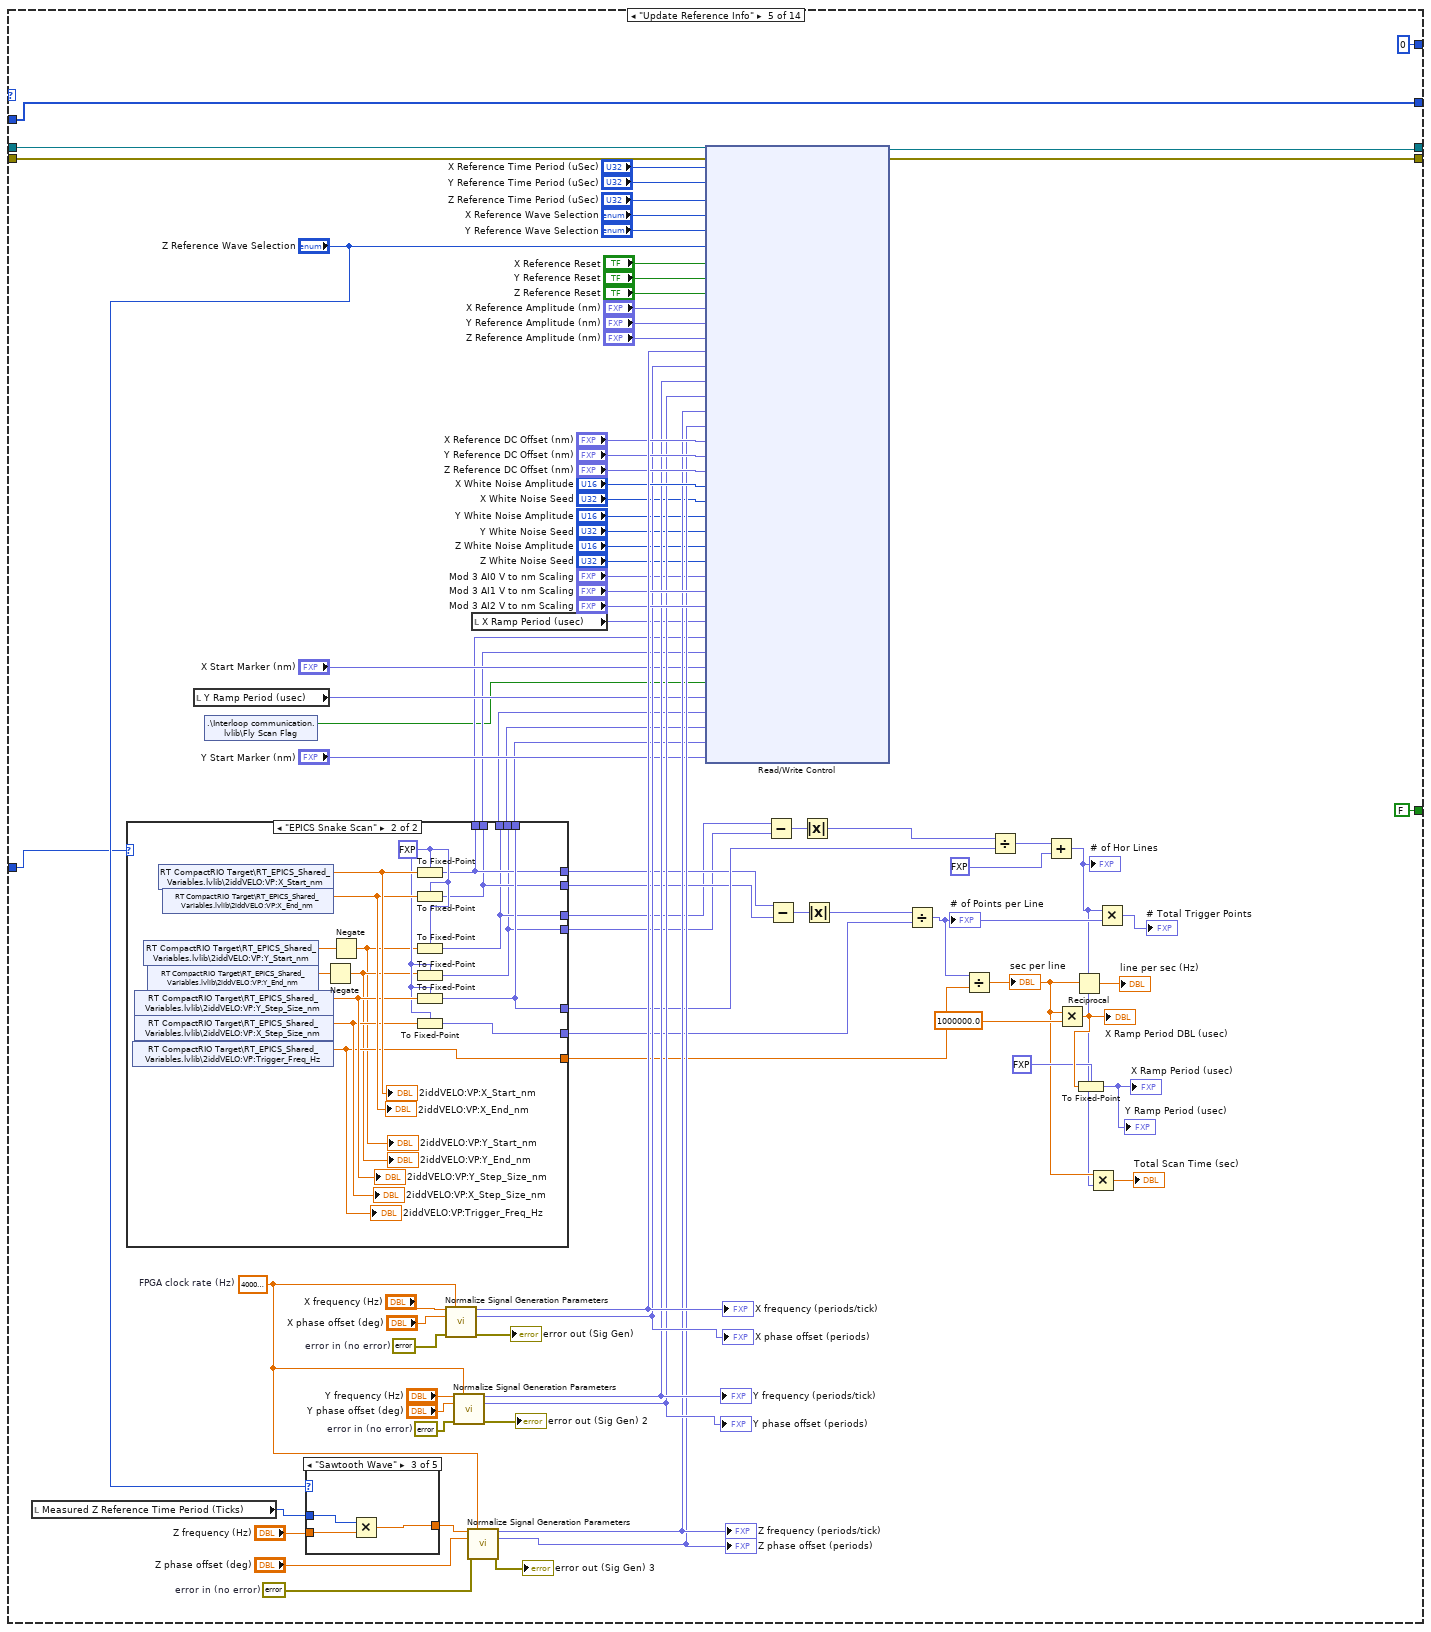
[diagram p20: hidden frame]
diagram:
  w3 = T12[] [enum."Initialization", enum."Import Controller coeffs", enum."Update Controller Info", enum."Wait"] items=["Initialization", "Import Controller coeffs", "Update Controller Info", "Wait", "Update Reference Info", "Update Detector Trigger Info", "Update Datalog Info", "Check FPGA Status", "Pre-Scan", "Start Scan", "Scanning", "End Scan", "Restart FPGA", "Stop FPGA"] ("Reduced Array of States")
  # "Epics command loop\n\nNeed to create enum PV for commands that replicate local\ncommand structure -- this will allow to update in PID mode\n\nShould make PV readback for scan type (Hinf-Fly/Hinf-Step/PID-Fly/PID-Step/\nOpen-FLy/Open-Step)"
  # "FPGA reference"
  # "Array of states to process"
  # "Next state to go to"
  n1 = flat-sequence {
    tunnel: [State_Enum."Initialization" ("States")] -> w4
    tunnel: [w16] -> w1
    tunnel: [w15] -> w2
    frame #0 {
      w10 = FALSE ("Start_Scan")
      w13 = "base_name" ("Base_Filename")
      # "Should add other PVs here for initialization"
      n2 = xnode ("Open FPGA VI Reference")("error in"=errorcluster {"status"=FALSE, "code"=0, "source"=""} ("error constant"), "resource name"=tag "rio://164.54.113.14/RIO0") -> ("FPGA VI Reference Out"=w15:refnum<k20>, "error out"=w16:errorcluster)
      n3 = shared-variable ".\\Interloop communication.lvlib\\Base Filename"(w13) -> ()  [unwired: 1 in, 1 out]
      n4 = shared-variable "RT CompactRIO Target\\RT_EPICS_Shared_Variables.lvlib\\2iddVELO:VP:Base_Filename"(w13) -> ()  [unwired: 1 in, 1 out]
      n5 = shared-variable "RT CompactRIO Target\\RT_EPICS_Shared_Variables.lvlib\\2iddVELO:VP:Remote_Scan"(TRUE ("Remote_Scan")) -> ()  [unwired: 1 in, 1 out]
      n6 = shared-variable "RT CompactRIO Target\\RT_EPICS_Shared_Variables.lvlib\\2iddVELO:VP:Fly_Scan"(FALSE ("Fly_Scan")) -> ()  [unwired: 1 in, 1 out]
      n7 = local write "Stop System (Careful!!)"(FALSE ("Stop")) -> ()
      n8 = shared-variable "RT CompactRIO Target\\RT_EPICS_Shared_Variables.lvlib\\2iddVELO:VP:Execute_Command"(w10) -> ()  [unwired: 1 in, 1 out]
      n9 = shared-variable "RT CompactRIO Target\\RT_EPICS_Shared_Variables.lvlib\\2iddVELO:VP:Scanning"(w10) -> ()  [unwired: 1 in, 1 out]
    }
  }
  n10 = node-c288() -> (w9:T14)  [unwired: 4 in]
  n11 = while {
    i -> [w20]
    stop <- w21 stop-if-true
    # "Command  Loop"
    n12 = Wait Until Next ms Multiple(millisecond multiple=u32 50) -> ()  [unwired: 1 out]
    n13 = case shown="False" "Stop System (Careful!!)" {
      tunnel: [FALSE TRUE] -> w21
      frame False {
        n14 = shared-variable "RT CompactRIO Target\\RT_EPICS_Shared_Variables.lvlib\\2iddVELO:VP:Remote_Scan"() -> (w32:bool, error out=w30:errorcluster)  [unwired: 1 in]
        n15 = shared-variable "RT CompactRIO Target\\RT_EPICS_Shared_Variables.lvlib\\2iddVELO:VP:Local_Lock"("Local_Lock", error in=w30) -> (error out=w24:errorcluster)
        n16 = shared-variable ".\\Interloop communication.lvlib\\New Command"() -> (w36:bool)  [unwired: 1 in, 1 out]
        n17 = Not(x="Local_Lock") -> (.not. x?=w27:bool)
        n18 = And(x=w32, y=w27) -> (x .and. y?=w33:bool)
        "Remote Mode" <- w33
        n19 = Not(x=w36) -> (.not. x?=w35:bool)
        n20 = case shown="True" w33 {
          tunnel: w35 -> [w48 w62]
          tunnel: [enum16{"FPGA Snake Scan", "EPICS Snake Scan"}."FPGA Snake Scan" ("Snake Scan Reference FPGA or EPICS") enum16{"FPGA Snake Scan", "EPICS Snake Scan"}."EPICS Snake Scan" ("Snake Scan Reference FPGA or EPICS")] -> w34
          tunnel: w24 -> [w41 w54]
          tunnel: [w43 w60] -> w29
          tunnel: ["Base name" w59] -> w26
          tunnel: [w38 w56] -> w25
          frame False {
            # "Running  in local mode"
            n21 = And(x="Execute", y=w48) -> (x .and. y?=w45:bool)
            n22 = case shown="True" w45 {
              frame False {
              }
              frame True {
                n23 = shared-variable ".\\Interloop communication.lvlib\\New Command"(TRUE ("New Command")) -> ()  [unwired: 1 in, 1 out]
                n24 = shared-variable ".\\Interloop communication.lvlib\\System command"("System command") -> ()  [unwired: 1 in, 1 out]
                n25 = local write "Execute"(FALSE ("Execute")) -> ()
              }
            }
            n26 = Equal?(x="Scan type", y=Scan_type."Fly" ("x")) -> (x = y?=w38:bool)
            n27 = Format Into String(error in=w41, "Scan type") -> (resulting string=w42:string, error out=w40:errorcluster)  [unwired: 2 in]
            n28 = shared-variable "RT CompactRIO Target\\RT_EPICS_Shared_Variables.lvlib\\2iddVELO:VP:Scan_Type"(w42, error in=w40) -> (error out=w43:errorcluster)
          }
          frame True {
            # "Running in remote mode via EPICS PVs"
            n29 = shared-variable "RT CompactRIO Target\\RT_EPICS_Shared_Variables.lvlib\\2iddVELO:VP:Execute_Command"(error in=w54) -> (w55:bool, error out=w53:errorcluster)
            "EPICS Execute Command" <- w55
            n30 = shared-variable "RT CompactRIO Target\\RT_EPICS_Shared_Variables.lvlib\\2iddVELO:VP:Base_Filename"() -> (w59:string)  [unwired: 1 in, 1 out]
            n31 = And(x=w62, y=w55) -> (x .and. y?=w61:bool)
            n32 = case shown="True" w61 {
              tunnel: [w64 w70] -> w60
              tunnel: w53 -> [w64 w67]
              frame False {
              }
              frame True {
                n33 = local read "EPICS cRIO Command"() -> (w68:T13)
                n34 = shared-variable "RT CompactRIO Target\\RT_EPICS_Shared_Variables.lvlib\\2iddVELO:VP:Execute_Command"(FALSE ("2iddVELO:VP:Flyscan_Start"), error in=w67) -> (error out=w70:errorcluster)
                n35 = local write "System Loop Type"(enum16{"Open Loop", "Closed Loop"}."Closed Loop" ("System Loop Type")) -> ()
                n36 = case shown="\"Reload Controller\"" w68 {
                  tunnel: [Command_Enum."Scan" ("System command") Command_Enum."Stop Scan" ("System command") Command_Enum."Re-Initialize " ("System command")] -> w65
                  frame "Start Scan", Default {
                  }
                  frame "Stop Scan" {
                  }
                  frame "Reload Controller" {
                  }
                }
                n37 = shared-variable ".\\Interloop communication.lvlib\\New Command"(TRUE ("New Command")) -> ()  [unwired: 1 in, 1 out]
                n38 = shared-variable ".\\Interloop communication.lvlib\\System command"(w65) -> ()  [unwired: 1 in, 1 out]
              }
            }
            n39 = local read "EPICS Scan Type"() -> (w57:T2)
            n40 = local write "Base name"(w59) -> ()
            n41 = Equal?(x=Scan_type."Fly", y=w57) -> (x = y?=w56:bool)
            n42 = local read "EPICS Controller Type"() -> (w52:T3)
            n43 = local write "Scan type"(w57) -> ()
            n44 = local write "Controller Type"(w52) -> ()
          }
        }
        "Snake Scan Reference FPGA or EPICS" <- w34
        "Command Loop Error" <- w29
        n45 = shared-variable ".\\Interloop communication.lvlib\\Base Filename"(w26) -> ()  [unwired: 1 in, 1 out]
        n46 = shared-variable ".\\Interloop communication.lvlib\\Fly Scan Flag"(w25) -> ()  [unwired: 1 in, 1 out]
        n47 = shared-variable ".\\Interloop communication.lvlib\\Command Loop Error"(w29) -> ()  [unwired: 1 in, 1 out]
      }
      frame True {
        n48 = shared-variable ".\\Interloop communication.lvlib\\System command"(Command_Enum."Stop System" ("System command")) -> (error out=w75:errorcluster)  [unwired: 1 in]
        n49 = shared-variable ".\\Interloop communication.lvlib\\New Command"(TRUE ("New Command"), error in=w75) -> ()  [unwired: 1 out]
      }
    }
    "Command Loop Iterations" <- w20
  }
  n50 = while {
    shift-right: [w92] -> _
    shift-left: TRUE -> [w93]
    i -> [w81]
    stop <- w85 stop-if-true
    # "Heartbeat Loop"
    n51 = shared-variable ".\\Interloop communication.lvlib\\EPICS command error"() -> (w79:errorcluster)  [unwired: 1 in, 1 out]
    n52 = shared-variable ".\\Interloop communication.lvlib\\Command Loop Error"() -> (w87:errorcluster)  [unwired: 1 in, 1 out]
    n53 = shared-variable ".\\Interloop communication.lvlib\\FPGA startup error"() -> (w84:errorcluster)  [unwired: 1 in, 1 out]
    n54 = Not(x=w93) -> (.not. x?=w92:bool)
    "Heartbeat" <- w92
    n55 = shared-variable ".\\Interloop communication.lvlib\\Readback Loop Error"() -> (w86:errorcluster)  [unwired: 1 in, 1 out]
    n56 = shared-variable ".\\Interloop communication.lvlib\\Main Loop Error"() -> (w91:errorcluster)  [unwired: 1 in, 1 out]
    n57 = call <vilib>:"RT LEDs.vi"("State"=3, "LED Num"=0) -> ("error out"=w80:errorcluster)  [unwired: 4 in, 1 out]
    n58 = Merge Errors(w80, w79, w87, w84, w91, w86) -> (w88:errorcluster)
    n59 = case shown="No Error" w88 {
      selector: w88 -> [w94 w96]
      tunnel: [u32 500 ("millisecond multiple") u32 100 ("millisecond multiple")] -> w90
      tunnel: [w94 w96] -> w89
      frame No Error {
      }
      frame Error {
      }
    }
    "RT error" <- w89
    n60 = local read "Stop System (Careful!!)"() -> (w85:bool)
    n61 = Wait Until Next ms Multiple(millisecond multiple=w90) -> ()  [unwired: 1 out]
    "Heartbeat Loop Iterations" <- w81
  }
  n62 = timed-loop {
    timing: w9 -> [_]
    timing-out: [_] -> w8
    shift-right: [w104] -> _
    shift-left: w4 -> [w98]
    shift-right: [w111] -> _
    shift-left: w2 -> [w105]
    shift-right: [w102] -> _
    shift-left: w1 -> [w106]
    shift-right: [w108] -> _
    shift-left: w3 -> [w109]
    i -> [w110]
    stop <- w113 stop-if-true
    # "Main Loop"
    n63 = node-c288() -> ()  [unwired: 1 in, 1 out]
    n64 = local read "Snake Scan Reference FPGA or EPICS"() -> (w103:enum16{"FPGA Snake Scan", "EPICS Snake Scan"})
    n65 = Format Into String(format string="%s", w98) -> (resulting string=w99:string)  [unwired: 2 in, 1 out]
    n66 = shared-variable "RT CompactRIO Target\\RT_EPICS_Shared_Variables.lvlib\\2iddVELO:VP:RT_State"(w99) -> ()  [unwired: 1 in, 1 out]
    n67 = case shown="\"Import Controller coeffs\"" w98 {
      tunnel: [w120 w140 w178 w235 w271 w386 w419 w432 w455 w496 w517 w577 w592 w604] -> w112
      tunnel: [FALSE ("Stop") FALSE ("Stop") FALSE ("Stop") FALSE ("Stop") FALSE ("Stop") FALSE ("Stop") FALSE ("Stop") FALSE ("Stop") _ FALSE ("Stop") FALSE ("Stop") FALSE ("Stop") FALSE ("Stop") TRUE ("Stop")] -> w113
      tunnel: [w123 w145 w177 w237 w269 w385 w418 w434 w446 w480 w543 w572 w587 w601] -> w111
      tunnel: [w115 w142 w176 w231 w268 w384 w417 w425 w445 w483 w541 w575 w586 w606] -> w102
      tunnel: w106 -> [w121 w137 w180 w232 w278 w388 w420 w435 w453 w481 w548 w567 w590 w610]
      tunnel: w105 -> [w122 w145 w179 w237 w279 w389 w421 w436 w454 w479 w544 w569 w596 w611]
      tunnel: w109 -> [w120 w140 w178 _ w271 w386 w419 w432 w455 w496 w518 w577 w592 _]
      tunnel: [i64 0 i64 0 i64 0 i64 50 i64 0 i64 0 i64 0 i64 0 i64 0 i64 250 w499 i64 0 i64 0 i64 0] -> w107
      tunnel: w103 -> [_ _ _ _ w265 w381 _ _ _ _ _ _ _ _]
      frame "Initialization", Default {
        n68 = xnode "Invoke Method"("FPGA VI Reference In"=w122, "error in"=w121, "Requested Depth"="Requested Depth") -> ("FPGA VI Reference Out"=w125:refnum<k20>, "error out"=w124:errorcluster, "Actual Depth"=→"Actual Depth":u32)
        n69 = xnode "Read/Write Control"("FPGA VI Reference In"=w125, "error in"=w124, "Datalog Time Period (uSec)"="Datalog Time Period (uSec)", "Datalog Cases"="Datalog Cases") -> ("FPGA VI Reference Out"=w117:refnum<k20>, "error out"=w116:errorcluster)
        n70 = xnode "Read/Write Control"("FPGA VI Reference In"=w117, "error in"=w116) -> ("FPGA VI Reference Out"=w123:refnum<k20>, "error out"=w115:errorcluster, "Wait error"=w114:errorcluster)
        "FPGA wait error" <- w114
        n71 = shared-variable ".\\Interloop communication.lvlib\\FPGA startup error"(w114) -> ()  [unwired: 1 in, 1 out]
      }
      frame "Import Controller coeffs" {
        n72 = case shown="\"PID\"" "Controller Type" {
          tunnel: ["file path soscoeff_xx1 Hinf" "file path soscoeff_xx1 PID"] -> w136
          tunnel: ["file path sos gain SF Controller_xx1 Hinf" "file path sos gain SF Controller_xx1 PID"] -> w135
          tunnel: ["file path soscoeff_yy1 Hinf" "file path soscoeff_yy1 PID"] -> w134
          tunnel: ["file path sos gain SF Controller_yy1 Hinf" "file path sos gain SF Controller_yy1 PID"] -> w133
          tunnel: ["file path sos gain SF Controller_zz1 Hinf" "file path sos gain SF Controller_zz1 PID"] -> w132
          tunnel: ["file path soscoeff_zz1 Hinf" "file path soscoeff_zz1 PID"] -> w131
          frame "H-infinity", Default {
          }
          frame "PID" {
          }
        }
        n73 = call "Read_coeff.vi"("error in (no error)"=w137, "sos gain SF controller file path"=w132, "sos coeff file path"=w131) -> ("b02(2)"=→"b02(2) zz1c":fxp<+/-,64,9>[], "b01(2)"=→"b01(2) zz1c":fxp<+/-,64,9>[], "-a02(2)"=→"-a02(2) zz1c":fxp<+/-,64,9>[], "-a01(2)"=→"-a01(2) zz1c":fxp<+/-,64,9>[], "error out"=w141:errorcluster, "sos gain SF Controller"=→"sos gain SF Controller zz1c":fxp<+/-,42,9>)  [unwired: 3 in]
        n74 = call "Read_coeff.vi"("error in (no error)"=w137, "sos gain SF controller file path"=w133, "sos coeff file path"=w134) -> ("b02(2)"=→"b02(2) yy1c":fxp<+/-,64,9>[], "b01(2)"=→"b01(2) yy1c":fxp<+/-,64,9>[], "-a02(2)"=→"-a02(2) yy1c":fxp<+/-,64,9>[], "-a01(2)"=→"-a01(2) yy1c":fxp<+/-,64,9>[], "error out"=w139:errorcluster, "sos gain SF Controller"=→"sos gain SF Controller yy1c":fxp<+/-,42,9>)  [unwired: 3 in]
        n75 = call "Read_coeff.vi"("error in (no error)"=w137, "sos gain SF controller file path"=w135, "sos coeff file path"=w136) -> ("b02(2)"=→"b02(2) xx1c":fxp<+/-,64,9>[], "b01(2)"=→"b01(2) xx1c":fxp<+/-,64,9>[], "-a02(2)"=→"-a02(2) xx1c":fxp<+/-,64,9>[], "-a01(2)"=→"-a01(2) xx1c":fxp<+/-,64,9>[], "error out"=w138:errorcluster, "sos gain SF Controller"=→"sos gain SF Controller xx1c":fxp<+/-,42,9>)  [unwired: 3 in]
        n76 = Merge Errors(w138, w139, w141) -> (w142:errorcluster)
        "Coeff file import error" <- w142
      }
      frame "Update Controller Info" {
        n77 = local read "sos gain SF Controller yy1c"() -> (w209:fxp<+/-,42,9>)
        n78 = local read "sos gain SF Controller xx1c"() -> (w214:fxp<+/-,42,9>)
        n79 = local read "sos gain SF Controller zz1c"() -> (w207:fxp<+/-,42,9>)
        n80 = local read "-a01(2) yy1c"() -> (w213:fxp<+/-,64,9>[])
        n81 = local read "-a02(2) yy1c"() -> (w212:fxp<+/-,64,9>[])
        n82 = local read "-a01(2) xx1c"() -> (w218:fxp<+/-,64,9>[])
        n83 = local read "-a02(2) xx1c"() -> (w217:fxp<+/-,64,9>[])
        n84 = local read "-a01(2) zz1c"() -> (w208:fxp<+/-,64,9>[])
        n85 = local read "-a02(2) zz1c"() -> (w204:fxp<+/-,64,9>[])
        n86 = local read "b01(2) yy1c"() -> (w211:fxp<+/-,64,9>[])
        n87 = local read "b02(2) yy1c"() -> (w210:fxp<+/-,64,9>[])
        n88 = local read "b01(2) xx1c"() -> (w216:fxp<+/-,64,9>[])
        n89 = local read "b02(2) xx1c"() -> (w215:fxp<+/-,64,9>[])
        n90 = local read "b01(2) zz1c"() -> (w205:fxp<+/-,64,9>[])
        n91 = local read "b02(2) zz1c"() -> (w206:fxp<+/-,64,9>[])
        n92 = Or(x="Optics Z Reset", y="Reset All") -> (x .or. y?=w198:bool)
        n93 = Or(x="Sample Z Reset", y="Reset All") -> (x .or. y?=w195:bool)
        n94 = Or(x="Optics X Reset", y="Reset All") -> (x .or. y?=w202:bool)
        n95 = Or(x="Optics Y Reset", y="Reset All") -> (x .or. y?=w200:bool)
        n96 = Or(x="Sample X Reset", y="Reset All") -> (x .or. y?=w197:bool)
        n97 = Or(x="Sample Y Reset", y="Reset All") -> (x .or. y?=w196:bool)
        n98 = xnode "Read/Write Control"("FPGA VI Reference In"=w179, "error in"=w180, "Wait timer (ms)"="FPGA Wait Timer (ms)", "Controller Time Period (uSec)"="Controller Time Period (uSec)", "Controller Output Time Period (uSec)"="Controller Output Time Period (uSec)", "System Loop Type"="System Loop Type", "Controller Output Upper Limit"="Controller Output Upper Limit", "Controller Output Lower Limit"="Controller Output Lower Limit", "X-Stage nm to V Scaling"="X-Stage nm to V Scaling", "X-Stage Scaling Direction"="X-Stage Scaling Direction", "Y-Stage nm to V Scaling"="Y-Stage nm to V Scaling", "Z-Stage nm to V Scaling"="Z-Stage nm to V Scaling", "Plant Output Time Period (uSec)"="Plant Output Time Period (uSec)", "Reset Optics X"=w202, "Reset Optics Y"=w200, "Reset Optics Z"=w198, "Reset Sample X"=w197, "Reset Sample Y"=w196, "Reset Sample Z"=w195, "Optics X Stage Resolution (nm)"="Optics X Stage Resolution (nm)", "Optics Y Stage Resolution (nm)"="Optics Y Stage Resolution (nm)", "Optics Z Stage Resolution (nm)"="Optics Z Stage Resolution (nm)", "Sample X Stage Resolution (nm)"="Sample X Stage Resolution (nm)", "Sample Y Stage Resolution (nm)"="Sample Y Stage Resolution (nm)", "Sample Z Stage Resolution (nm)"="Sample Z Stage Resolution (nm)", "Scaling mV to V"="Scaling mV to V", "-a01(2) xx1"=w218, "-a02(2) xx1"=w217, "b01(2) xx1"=w216, "b02(2) xx1"=w215, "sos gain SF Controller xx1"=w214, "-a01(2) yy1"=w213, "-a02(2) yy1"=w212, "b01(2) yy1"=w211, "b02(2) yy1"=w210, "sos gain SF Controller yy1"=w209, "-a01(2) zz1"=w208, "-a02(2) zz1"=w204, "b01(2) zz1"=w205, "b02(2) zz1"=w206, "sos gain SF Controller zz1"=w207, "Analog Input Time Period (uSec)"="Analog Input Time Period (uSec)", "Optics and or Sample Stage"="Optics and or Sample Stage", "Y-Stage Scaling Direction"="Y-Stage Scaling Direction", "Z-Stage Scaling Direction"="Z-Stage Scaling Direction") -> ("FPGA VI Reference Out"=w177:refnum<k20>, "error out"=w176:errorcluster)
      }
      frame "Wait" {
        n99 = shared-variable ".\\Interloop communication.lvlib\\New Command"() -> (w236:bool, error out=w234:errorcluster)  [unwired: 1 in]
        n100 = case shown="True" w236 {
          tunnel: [w239 w240] -> w235
          tunnel: w234 -> [_ w244]
          tunnel: w232 -> [w238 w242]
          tunnel: [w238 w241] -> w231
          frame False {
            w239 = T12[] [enum."Wait"] items=["Initialization", "Import Controller coeffs", "Update Controller Info", "Wait", "Update Reference Info", "Update Detector Trigger Info", "Update Datalog Info", "Check FPGA Status", "Pre-Scan", "Start Scan", "Scanning", "End Scan", "Restart FPGA", "Stop FPGA"]
          }
          frame True {
            n101 = shared-variable ".\\Interloop communication.lvlib\\System command"() -> (w243:T9)  [unwired: 1 in, 1 out]
            "Last Command Executed" <- w243
            n102 = case shown="\"Stop Scan\"" w243 {
              tunnel: [w248 w251 w254 w257 w260 w264] -> w240
              tunnel: w242 -> [w247 w250 w253 w256 w259 w263]
              tunnel: [w246 w249 w252 w255 w258 w262] -> w241
              frame "Re-Initialize ", Default {
                w248 = T12[] [enum."Initialization", enum."Import Controller coeffs", enum."Update Controller Info", enum."Wait"] items=["Initialization", "Import Controller coeffs", "Update Controller Info", "Wait", "Update Reference Info", "Update Detector Trigger Info", "Update Datalog Info", "Check FPGA Status", "Pre-Scan", "Start Scan", "Scanning", "End Scan", "Restart FPGA", "Stop FPGA"]
                n103 = call <vilib>:"Clear Errors.vi"("error in (no error)"=w247) -> ("error out"=w246:errorcluster)  [unwired: 5 in, 1 out]
              }
              frame "Update Scan Settings" {
                w251 = T12[] [enum."Update Reference Info", enum."Update Detector Trigger Info", enum."Update Datalog Info", enum."Wait"] items=["Initialization", "Import Controller coeffs", "Update Controller Info", "Wait", "Update Reference Info", "Update Detector Trigger Info", "Update Datalog Info", "Check FPGA Status", "Pre-Scan", "Start Scan", "Scanning", "End Scan", "Restart FPGA", "Stop FPGA"]
                n104 = call <vilib>:"Clear Errors.vi"("error in (no error)"=w250) -> ("error out"=w249:errorcluster)  [unwired: 5 in, 1 out]
              }
              frame "Scan" {
                w254 = T12[] [enum."Update Reference Info", enum."Update Detector Trigger Info", enum."Update Datalog Info", enum."Pre-Scan", enum."Start Scan", enum."Scanning", enum."End Scan", enum."Wait"] items=["Initialization", "Import Controller coeffs", "Update Controller Info", "Wait", "Update Reference Info", "Update Detector Trigger Info", "Update Datalog Info", "Check FPGA Status", "Pre-Scan", "Start Scan", "Scanning", "End Scan", "Restart FPGA", "Stop FPGA"]
                n105 = call <vilib>:"Clear Errors.vi"("error in (no error)"=w253) -> ("error out"=w252:errorcluster)  [unwired: 5 in, 1 out]
              }
              frame "Stop Scan" {
                w257 = T12[] [enum."End Scan", enum."Wait"] items=["Initialization", "Import Controller coeffs", "Update Controller Info", "Wait", "Update Reference Info", "Update Detector Trigger Info", "Update Datalog Info", "Check FPGA Status", "Pre-Scan", "Start Scan", "Scanning", "End Scan", "Restart FPGA", "Stop FPGA"]
                n106 = call <vilib>:"Clear Errors.vi"("error in (no error)"=w256) -> ("error out"=w255:errorcluster)  [unwired: 5 in, 1 out]
              }
              frame "Restart FPGA" {
                w260 = T12[] [enum."Restart FPGA", enum."Initialization", enum."Import Controller coeffs", enum."Update Controller Info", enum."Wait"] items=["Initialization", "Import Controller coeffs", "Update Controller Info", "Wait", "Update Reference Info", "Update Detector Trigger Info", "Update Datalog Info", "Check FPGA Status", "Pre-Scan", "Start Scan", "Scanning", "End Scan", "Restart FPGA", "Stop FPGA"]
                n107 = call <vilib>:"Clear Errors.vi"("error in (no error)"=w259) -> ("error out"=w258:errorcluster)  [unwired: 5 in, 1 out]
              }
              frame "Stop System" {
                w264 = T12[] [enum."Stop FPGA"] items=["Initialization", "Import Controller coeffs", "Update Controller Info", "Wait", "Update Reference Info", "Update Detector Trigger Info", "Update Datalog Info", "Check FPGA Status", "Pre-Scan", "Start Scan", "Scanning", "End Scan", "Restart FPGA", "Stop FPGA"]
                n108 = call <vilib>:"Clear Errors.vi"("error in (no error)"=w263) -> ("error out"=w262:errorcluster)  [unwired: 5 in, 1 out]
                n109 = local write "Stop System (Careful!!)"(TRUE ("Stop")) -> ()
              }
            }
            n110 = shared-variable ".\\Interloop communication.lvlib\\New Command"(FALSE ("New Command"), error in=w244) -> ()  [unwired: 1 out]
          }
        }
      }
      frame "Update Reference Info" {
        w331 = errorcluster {"status"=FALSE, "code"=0, "source"=""}  # error in (no error)
        w334 = errorcluster {"status"=FALSE, "code"=0, "source"=""}  # error in (no error)
        w348 = errorcluster {"status"=FALSE, "code"=0, "source"=""}  # error in (no error)
        w327 = 40000000.0  # FPGA clock rate (Hz)
        n111 = local read "Measured Z Reference Time Period (Ticks)"() -> (w270:u32)
        n112 = case shown="\"EPICS Snake Scan\"" w265 {
          tunnel: ["X Ramp Start (nm)" w364] -> w286
          tunnel: ["X Ramp End (nm)" w363] -> w285
          tunnel: ["Y Ramp Start (nm)" w362] -> w284
          tunnel: ["Y Ramp End (nm)" w361] -> w283
          tunnel: ["Y Step Size (nm)" w365] -> w282
          tunnel: ["X Step Size (nm)" w368] -> w281
          tunnel: [w356 w366] -> w280
          tunnel: ["Y Step Size (nm)" w365] -> w277
          tunnel: ["X Ramp Start (nm)" w364] -> w276
          tunnel: ["X Ramp End (nm)" w363] -> w275
          tunnel: ["Y Ramp Start (nm)" w362] -> w274
          tunnel: ["Y Ramp End (nm)" w361] -> w273
          frame "FPGA Snake Scan", Default {
            n113 = local read "DT Frequency (Hz)"() -> (w356:dbl)
          }
          frame "EPICS Snake Scan" {
            w367 = fxp<+/-,16,16> 0.0 ("fixed-point type")
            n114 = shared-variable "RT CompactRIO Target\\RT_EPICS_Shared_Variables.lvlib\\2iddVELO:VP:Trigger_Freq_Hz"() -> (w366:dbl)  [unwired: 1 in, 1 out]
            "2iddVELO:VP:Trigger_Freq_Hz" <- w366
            n115 = shared-variable "RT CompactRIO Target\\RT_EPICS_Shared_Variables.lvlib\\2iddVELO:VP:Y_Step_Size_nm"() -> (w370:dbl)  [unwired: 1 in, 1 out]
            "2iddVELO:VP:Y_Step_Size_nm" <- w370
            n116 = shared-variable "RT CompactRIO Target\\RT_EPICS_Shared_Variables.lvlib\\2iddVELO:VP:X_Step_Size_nm"() -> (w369:dbl)  [unwired: 1 in, 1 out]
            "2iddVELO:VP:X_Step_Size_nm" <- w369
            n117 = shared-variable "RT CompactRIO Target\\RT_EPICS_Shared_Variables.lvlib\\2iddVELO:VP:Y_Start_nm"() -> (w371:dbl)  [unwired: 1 in, 1 out]
            n118 = shared-variable "RT CompactRIO Target\\RT_EPICS_Shared_Variables.lvlib\\2iddVELO:VP:Y_End_nm"() -> (w360:dbl)  [unwired: 1 in, 1 out]
            n119 = shared-variable "RT CompactRIO Target\\RT_EPICS_Shared_Variables.lvlib\\2iddVELO:VP:X_Start_nm"() -> (w373:dbl)  [unwired: 1 in, 1 out]
            "2iddVELO:VP:X_Start_nm" <- w373
            n120 = shared-variable "RT CompactRIO Target\\RT_EPICS_Shared_Variables.lvlib\\2iddVELO:VP:X_End_nm"() -> (w372:dbl)  [unwired: 1 in, 1 out]
            "2iddVELO:VP:X_End_nm" <- w372
            n121 = Negate(x=w360) -> (-x=w359:dbl)
            "2iddVELO:VP:Y_End_nm" <- w359
            n122 = Negate(x=w371) -> (-x=w358:dbl)
            "2iddVELO:VP:Y_Start_nm" <- w358
            n123 = To Fixed-Point(fixed-point type=w367, number=w373) -> (fixed-point=w364:fxp<+/-,16,16>)
            n124 = To Fixed-Point(fixed-point type=w367, number=w372) -> (fixed-point=w363:fxp<+/-,16,16>)
            n125 = To Fixed-Point(fixed-point type=w367, number=w358) -> (fixed-point=w362:fxp<+/-,16,16>)
            n126 = To Fixed-Point(fixed-point type=w367, number=w359) -> (fixed-point=w361:fxp<+/-,16,16>)
            n127 = To Fixed-Point(fixed-point type=w367, number=w370) -> (fixed-point=w365:fxp<+/-,16,16>)
            n128 = To Fixed-Point(fixed-point type=w367, number=w369) -> (fixed-point=w368:fxp<+/-,16,16>)
          }
        }
        n129 = local read "Y Ramp Period (usec)"() -> (w288:fxp<+,24,24>)
        n130 = shared-variable ".\\Interloop communication.lvlib\\Fly Scan Flag"() -> (w272:bool)  [unwired: 1 in, 1 out]
        n131 = case shown="\"Sawtooth Wave\"" "Z Reference Wave Selection" {
          tunnel: "Z frequency (Hz)" -> [w374 w375 w377 w379 w380]
          tunnel: [w374 w375 w376 w379 w380] -> w309
          tunnel: w270 -> [_ _ w378 _ _]
          frame "Constant", Default {
          }
          frame "Sine Wave" {
          }
          frame "Sawtooth Wave" {
            n132 = Multiply(x=w378, y=w377) -> (x*y=w376:dbl)
          }
          frame "Square Wave" {
          }
          frame "Filtered White Noise" {
          }
        }
        n133 = call <vilib>:"Normalize Signal Generation Parameters.vi"("frequency (Hz)"="X frequency (Hz)", "FPGA clock rate (Hz)"=w327, "phase offset (deg)"="X phase offset (deg)", "error in (no error)"=w348) -> ("frequency (periods/tick)"=w347:fxp<+,32,0>, "phase offset (periods)"=w337:fxp<+,32,0>, "error out"=→"error out (Sig Gen)":errorcluster)  [unwired: 6 in, 3 out]
        "X frequency (periods/tick)" <- w347
        "X phase offset (periods)" <- w337
        n134 = call <vilib>:"Normalize Signal Generation Parameters.vi"("frequency (Hz)"="Y frequency (Hz)", "FPGA clock rate (Hz)"=w327, "phase offset (deg)"="Y phase offset (deg)", "error in (no error)"=w334) -> ("frequency (periods/tick)"=w330:fxp<+,32,0>, "phase offset (periods)"=w329:fxp<+,32,0>, "error out"=→"error out (Sig Gen) 2":errorcluster)  [unwired: 6 in, 3 out]
        "Y frequency (periods/tick)" <- w330
        "Y phase offset (periods)" <- w329
        n135 = call <vilib>:"Normalize Signal Generation Parameters.vi"("frequency (Hz)"=w309, "FPGA clock rate (Hz)"=w327, "phase offset (deg)"="Z phase offset (deg)", "error in (no error)"=w331) -> ("frequency (periods/tick)"=w328:fxp<+,32,0>, "phase offset (periods)"=w320:fxp<+,32,0>, "error out"=→"error out (Sig Gen) 3":errorcluster)  [unwired: 6 in, 3 out]
        "Z frequency (periods/tick)" <- w328
        "Z phase offset (periods)" <- w320
        n136 = local read "X Ramp Period (usec)"() -> (w287:fxp<+,24,24>)
        n137 = xnode "Read/Write Control"("FPGA VI Reference In"=w279, "error in"=w278, "X Reference Time Period (uSec)"="X Reference Time Period (uSec)", "Y Reference Time Period (uSec)"="Y Reference Time Period (uSec)", "Z Reference Time Period (uSec)"="Z Reference Time Period (uSec)", "X Reference Wave Selection"="X Reference Wave Selection", "Y Reference Wave Selection"="Y Reference Wave Selection", "Z Reference Wave Selection"="Z Reference Wave Selection", "X Reference Reset"="X Reference Reset", "Y Reference Reset"="Y Reference Reset", "Z Reference Reset"="Z Reference Reset", "X Reference Amplitude (nm)"="X Reference Amplitude (nm)", "Y Reference Amplitude (nm)"="Y Reference Amplitude (nm)", "Z Reference Amplitude (nm)"="Z Reference Amplitude (nm)", "X Frequency (periods/tick)"=w347, "X Phase Offset (periods)"=w337, "Y Frequency (periods/tick)"=w330, "Y Phase Offset (periods)"=w329, "Z Frequency (periods/tick)"=w328, "Z Phase Offset (periods)"=w320, "X Reference DC Offset (nm)"="X Reference DC Offset (nm)", "Y Reference DC Offset (nm)"="Y Reference DC Offset (nm)", "Z Reference DC Offset (nm)"="Z Reference DC Offset (nm)", "X White Noise Amplitude"="X White Noise Amplitude", "X White Noise Seed"="X White Noise Seed", "Y White Noise Amplitude"="Y White Noise Amplitude", "Y White Noise Seed"="Y White Noise Seed", "Z White Noise Amplitude"="Z White Noise Amplitude", "Z White Noise Seed"="Z White Noise Seed", "Mod 3 AI0 V to nm Scaling"="Mod 3 AI0 V to nm Scaling", "Mod 3 AI1 V to nm Scaling"="Mod 3 AI1 V to nm Scaling", "Mod 3 AI2 V to nm Scaling"="Mod 3 AI2 V to nm Scaling", "X Ramp Period (usec)"=w287, "X Ramp Start (nm)"=w286, "X Ramp End (nm)"=w285, "X Start Marker (nm)"="X Start Marker (nm)", "Fly Scan"=w272, "Y Ramp Period (usec)"=w288, "Y Ramp Start (nm)"=w284, "Y Ramp End (nm)"=w283, "Y Ramp Drop Size (nm)"=w282, "Y Start Marker (nm)"="Y Start Marker (nm)") -> ("FPGA VI Reference Out"=w269:refnum<k20>, "error out"=w268:errorcluster)
        n138 = Subtract(x=w274, y=w273) -> (x-y=w304:fxp<+/-,17,17>)
        n139 = Subtract(x=w276, y=w275) -> (x-y=w302:fxp<+/-,17,17>)
        n140 = Absolute Value(x=w304) -> (abs(x)=w295:fxp<+,16,16>)
        n141 = Absolute Value(x=w302) -> (abs(x)=w301:fxp<+,16,16>)
        n142 = Divide(x=w301, y=w281) -> (x/y=w299:fxp<+/-,33,17>)
        "# of Points per Line" <- w299
        n143 = Divide(x=w299, y=w280) -> (x/y=w291:dbl)
        "sec per line" <- w291
        n144 = Divide(x=w295, y=w277) -> (x/y=w296:fxp<+/-,33,17>)
        n145 = Add(x=w296, y=fxp<+,16,16> 1.0) -> (x+y=w290:fxp<+/-,34,18>)
        "# of Hor Lines" <- w290
        n146 = Multiply(x=w291, y=1000000.0) -> (x*y=w294:dbl)
        "X Ramp Period DBL (usec)" <- w294
        n147 = Reciprocal(x=w291) -> (1/x=→"line per sec (Hz)":dbl)
        n148 = To Fixed-Point(fixed-point type=fxp<+,24,24> 0.0, number=w294) -> (fixed-point=→"X Ramp Period (usec)" →"Y Ramp Period (usec)":fxp<+,24,24>)
        n149 = Multiply(x=w291, y=w290) -> (x*y=→"Total Scan Time (sec)":dbl)
        n150 = Multiply(x=w290, y=w299) -> (x*y=→"# Total Trigger Points":fxp<+/-,64,34>)
      }
      frame "Update Detector Trigger Info" {
        w395 = 40000000.0  # FPGA clock rate (Hz)
        w397 = errorcluster {"status"=FALSE, "code"=0, "source"=""}  # error in (no error)
        n151 = case shown="\"EPICS Snake Scan\"" w381 {
          tunnel: ["DT Frequency (Hz)" w414] -> w396
          tunnel: ["DT duty cycle (%)" w413] -> w390
          frame "FPGA Snake Scan", Default {
          }
          frame "EPICS Snake Scan" {
            n152 = shared-variable "RT CompactRIO Target\\RT_EPICS_Shared_Variables.lvlib\\2iddVELO:VP:Trig_DutyCycle_Per"() -> (w413:dbl)  [unwired: 1 in, 1 out]
            "2iddVELO:VP:Trig_DutyCycle_Per" <- w413
            n153 = shared-variable "RT CompactRIO Target\\RT_EPICS_Shared_Variables.lvlib\\2iddVELO:VP:Trigger_Freq_Hz"() -> (w414:dbl)  [unwired: 1 in, 1 out]
          }
        }
        "Trigger Frequency (Hz)" <- w396
        "Trigger Duty Cycle (%)" <- w390
        n154 = call <vilib>:"Normalize Signal Generation Parameters.vi"("frequency (Hz)"=w396, "FPGA clock rate (Hz)"=w395, "phase offset (deg)"="DT phase offset (deg)", "duty cycle (%)"=w390, "error in (no error)"=w397) -> ("frequency (periods/tick)"=w393:fxp<+,32,0>, "phase offset (periods)"=w392:fxp<+,32,0>, "duty cycle (periods)"=w391:fxp<+,32,0>, "error out"=→"error out (Sig Gen) 4":errorcluster)  [unwired: 5 in, 2 out]
        "DT Frequency (periods/tick)" <- w393
        "DT Phase Offset (periods)" <- w392
        "DT Duty Cycle (periods)" <- w391
        n155 = xnode "Read/Write Control"("FPGA VI Reference In"=w389, "error in"=w388, "Detector Trigger Time Period (uSec)"="Detector Trigger Time Period (uSec)", "Trigger Generation Time Period (uSec)"="Trigger Generation Time Period (uSec)", "Detector Trigger Lower Limit (V)"="Detector Trigger Lower Limit (V)", "Detector Trigger Upper Limit (V)"="Detector Trigger Upper Limit (V)", "Trigger High Period (usec)"="Trigger High Period (usec)", "Trigger Low Period (usec)"="Trigger Low Period (usec)", "Trigger High Level (V)"="Trigger High Level (V)", "Trigger Low Level (V)"="Trigger Low Level (V)", "Trigger Wave Generator"="Trigger Wave Generator", "DT Reference Amplitude (V)"="DT Reference Amplitude (V)", "DT Reference DC Offset (V)"="DT Reference DC Offset (V)", "DT Frequency (periods/tick)"=w393, "DT Phase Offset (periods)"=w392, "DT Reset"="DT Reset", "DT Duty Cycle (periods)"=w391, "Data Trigger Time Period (uSec)"="Data Trigger Time Period (uSec)") -> ("FPGA VI Reference Out"=w385:refnum<k20>, "error out"=w384:errorcluster)
      }
      frame "Update Datalog Info" {
        n156 = local read "Datalog Time Period (uSec)"() -> (w424:u32)
        n157 = local read "Datalog Cases"() -> (w423:T4)
        n158 = xnode "Read/Write Control"("FPGA VI Reference In"=w421, "error in"=w420, "Datalog Time Period (uSec)"=w424, "Datalog Cases"=w423, "Timeout FPGA FIFO1"="Timeout FPGA FIFO1") -> ("FPGA VI Reference Out"=w418:refnum<k20>, "error out"=w417:errorcluster)
      }
      frame "Check FPGA Status" {
        n159 = xnode "Read/Write Control"("FPGA VI Reference In"=w436, "error in"=w435) -> ("FPGA VI Reference Out"=w434:refnum<k20>, "error out"=w433:errorcluster, "FPGA error monitor"=w439:errorcluster, "End Run Error"=w438:errorcluster, "FIFO Timed Out?"=→"FIFO Timed Out?":bool, "stop case"=w428:bool, "FIFO Timed Out"=w429:bool)
        "FPGA error monitor" <- w439
        "FPGA end run error" <- w438
        "stop case" <- w428
        "FIFO Timed Out" <- w429
        n160 = case shown="True" w428 {
          tunnel: [errorcluster {"status"=FALSE, "code"=0, "source"=""} ("error constant") errorcluster {"status"=TRUE, "code"=7002, "source"="FPGA stop case encountered"} ("error constant")] -> w426
          frame False {
          }
          frame True {
          }
        }
        n161 = case shown="True" w429 {
          tunnel: [errorcluster {"status"=FALSE, "code"=0, "source"=""} ("error constant") errorcluster {"status"=TRUE, "code"=7001, "source"="FPGA FIFO timed out"} ("error constant")] -> w427
          frame False {
          }
          frame True {
          }
        }
        n162 = Merge Errors(w433, w439, w438, w426, w427) -> (w425:errorcluster)
      }
      frame "Pre-Scan" {
        n163 = flat-sequence {
          tunnel: w454 -> [w461]
          tunnel: w453 -> [w460]
          tunnel: [w457] -> w452
          tunnel: [w456] -> w450
          tunnel: w452 -> [w467]
          tunnel: [w467] -> w451
          tunnel: w450 -> [w466]
          tunnel: [w466] -> w449
          tunnel: w451 -> [w471]
          tunnel: w449 -> [w470]
          tunnel: [w469] -> w448
          tunnel: [w468] -> w447
          tunnel: w448 -> [w478]
          tunnel: w447 -> [w477]
          tunnel: [w474] -> w446
          tunnel: [w473] -> w445
          frame #0 {
            w458 = TRUE
            n164 = xnode "Read/Write Control"("FPGA VI Reference In"=w461, "error in"=w460, "Reset Optics X"=w458, "Reset Optics Y"=w458, "Reset Optics Z"=w458, "Reset Sample X"=w458, "Reset Sample Y"=w458, "Reset Sample Z"=w458, "System Loop Type"=enum16{"Open Loop", "Closed Loop"}."Open Loop", "New FPGA command"=TRUE, "FPGA command"=enum16{"Start Scan", "Shutdown"}."Start Scan", "Fly Scan"=FALSE) -> ("FPGA VI Reference Out"=w457:refnum<k20>, "error out"=w456:errorcluster)
          }
          frame #1 {
            n165 = Wait (ms)(milliseconds to wait="Pre-Scan pause (ms)") -> ()  [unwired: 1 out]
          }
          frame #2 {
            n166 = xnode "Read/Write Control"("FPGA VI Reference In"=w471, "error in"=w470, "stop case"=TRUE) -> ("FPGA VI Reference Out"=w469:refnum<k20>, "error out"=w468:errorcluster)
          }
          frame #3 {
            w475 = FALSE ("Reset Optics X")
            # "Add Step vs FLy scan write here"
            n167 = local read "System Loop Type"() -> (w476:enum16{"Open Loop", "Closed Loop"})
            n168 = xnode "Read/Write Control"("FPGA VI Reference In"=w478, "error in"=w477, "Reset Optics X"=w475, "Reset Optics Y"=w475, "Reset Optics Z"=w475, "Reset Sample X"=w475, "Reset Sample Y"=w475, "Reset Sample Z"=w475, "System Loop Type"=w476) -> ("FPGA VI Reference Out"=w474:refnum<k20>, "error out"=w473:errorcluster)
          }
        }
      }
      frame "Start Scan" {
        n169 = shared-variable ".\\Interloop communication.lvlib\\Base Filename"() -> (w484:string)  [unwired: 1 in, 1 out]
        n170 = String To Path(string="cRIO data dir") -> (path=w485:path)
        "cRIO path" <- w485
        n171 = call "Data_Write.vi"("Destination dir"=w485, "error initialize"=w481, "Base name"=w484, "Command List"=Data_Write_Control."Initialize") -> ("error out"=w482:errorcluster, "Path"=w493:path)  [unwired: 4 in]
        n172 = Strip Path(path=w493) -> (stripped path=→"Output path":path, name=→"Output filename":string)
        n173 = shared-variable ".\\Interloop communication.lvlib\\Fly Scan Flag"() -> (w488:bool)  [unwired: 1 in, 1 out]
        n174 = xnode "Read/Write Control"("FPGA VI Reference In"=w479, "error in"=w482, "New FPGA command"=TRUE, "FPGA command"=enum16{"Start Scan", "Shutdown"}."Start Scan", "Fly Scan"=w488) -> ("FPGA VI Reference Out"=w480:refnum<k20>, "error out"=w483:errorcluster)
        n175 = shared-variable "RT CompactRIO Target\\RT_EPICS_Shared_Variables.lvlib\\2iddVELO:VP:Scanning"(w488) -> ()  [unwired: 1 in, 1 out]
      }
      frame "Scanning" {
        w539 = "%8f"  # format string
        w538 = ","  # delimiter (Tab)
        w556 = 0.0  # t0
        # "This creates time gap between subsequent\n reads in order to fill FIFO"
        n176 = xnode "Read/Write Control"("FPGA VI Reference In"=w544, "error in"=w548) -> ("FPGA VI Reference Out"=w529:refnum<k20>, "error out"=w528:errorcluster, "Number of Data Strings"=→"Number of Data Strings":i32, "FPGA state"=w523:T11)
        n177 = local read "Datalog Time Period (uSec)"() -> (w554:u32)
        n178 = Not Equal?(x=T11."Run", y=w523) -> (x != y?=w520:bool)
        n179 = Multiply(x=1e-06, y=w554) -> (x*y=w551:dbl)
        "Datalog Time Period (sec)" <- w551
        n180 = local read "Trigger Frequency (Hz)"() -> (w503:dbl)
        n181 = xnode "Invoke Method"("FPGA VI Reference In"=w529, "error in"=w528, "Number of Elements"=u32 0, "Timeout (ms)"=0) -> ("FPGA VI Reference Out"=w526:refnum<k20>, "error out"=w527:errorcluster, "Elements Remaining"=w507:u32)  [unwired: 1 out]
        n182 = Divide(x=1.0, y=w551) -> (x/y=w532:dbl)
        "Datalog Rate (Hz)" <- w532
        n183 = Multiply(x="FIFO Time Period", y=w532) -> (x*y=w504:dbl)
        n184 = Multiply(x=w504, y=5 ("Number of Data Strings 2")) -> (x*y=w530:dbl)
        n185 = To Unsigned Long Integer(number=w530) -> (unsigned 32bit integer=w525:u32)
        "Number of Elements" <- w525
        n186 = Divide(x=w503, y=w504) -> (x/y=w502:dbl)
        n187 = Divide(x=i16 1000, y=w502) -> (x/y=w500:dbl)
        n188 = Max & Min(x=w507, y=w525) -> (min(x,y)=w506:u32)  [unwired: 1 out]
        "Elements Available in FIFO" <- w506
        n189 = Equal?(x=u32 0, y=w507) -> (x = y?=w521:bool)
        n190 = And(x=w520, y=w521) -> (x .and. y?=w519:bool)
        n191 = xnode "Invoke Method"("FPGA VI Reference In"=w526, "error in"=w527, "Number of Elements"=w506, "Timeout (ms)"="Timeout (ms)") -> ("FPGA VI Reference Out"=w543:refnum<k20>, "error out"=w542:errorcluster, "Data"=w550:fxp<+/-,58,25>[], "Elements Remaining"=→"Elements Remaining" →"Elements Remaining in FIFO":u32)
        "Data" <- w550
        n192 = To Quad Integer(1:w500) -> (0:w499:i64)
        n193 = Decimate 1D Array(w550) -> (w515:fxp<+/-,58,25>[], w514:fxp<+/-,58,25>[], w513:fxp<+/-,58,25>[], w512:fxp<+/-,58,25>[], w545:fxp<+/-,58,25>[])
        n194 = Build Array(w515, w514, w513, w512, w545) -> (w557:fxp<+/-,58,25>[][])
        n195 = To Double Precision Float(number=w557) -> (double precision float=w552:dbl[][])
        n196 = Transpose 2D Array(2D array=w552) -> (transposed array=w547:dbl[][])
        n197 = case shown="True" w519 {
          tunnel: w518 -> [w562 w563]
          tunnel: [w560 w563] -> w517
          frame False {
            # "Either FIFO not empty or FPGA not \ndone running -- repeat scanning state"
            n198 = Insert Into Array(array=w562, index=0, new element=State_Enum."Scanning" ("new element/subarray")) -> (w560:T12[])
          }
          frame True {
            # "FIFO empty, FPGA done running \n-- moving onto next state"
          }
        }
        n199 = To Double Precision Float(number=w515) -> (double precision float=w511:dbl[])
        n200 = To Double Precision Float(number=w514) -> (double precision float=w510:dbl[])
        n201 = To Double Precision Float(number=w513) -> (double precision float=w509:dbl[])
        n202 = To Double Precision Float(number=w512) -> (double precision float=w508:dbl[])
        n203 = Bundle("t0"=w556, w551, w552) -> (→"Reference and Actual positions":cluster{"t0":dbl, dbl, dbl[][]})  [unwired: 1 in]
        n204 = Bundle(w509, w508) -> (→"XY actual":cluster{dbl[], dbl[]})  [unwired: 1 in]
        n205 = Bundle(w511, w510) -> (→"XY Ref":cluster{dbl[], dbl[]})  [unwired: 1 in]
        n206 = Array To Spreadsheet String(delimiter (Tab)=w538, array=w547, 3:w539) -> (spreadsheet string=w537:string)
        n207 = call "Data_Write.vi"("error initialize"=w548, "Data"=w537, "Command List"=Data_Write_Control."Write") -> ("error out"=w536:errorcluster)  [unwired: 5 in, 1 out]
        n208 = Merge Errors(w542, w536) -> (w541:errorcluster)
      }
      frame "End Scan" {
        n209 = xnode "Invoke Method"("FPGA VI Reference In"=w569, "error in"=w567) -> ("FPGA VI Reference Out"=w568:refnum<k20>, "error out"=w566:errorcluster)
        n210 = xnode "Read/Write Control"("FPGA VI Reference In"=w568, "error in"=w566, "stop case"=TRUE ("New FPGA command")) -> ("FPGA VI Reference Out"=w572:refnum<k20>, "error out"=w571:errorcluster)
        n211 = shared-variable "RT CompactRIO Target\\RT_EPICS_Shared_Variables.lvlib\\2iddVELO:VP:Scanning"(FALSE ("2iddVELO:VP:Fly_Scanning")) -> ()  [unwired: 1 in, 1 out]
        n212 = call "Data_Write.vi"("error initialize"=w571, "Command List"=Data_Write_Control."Close") -> ("error out"=w565:errorcluster)  [unwired: 6 in, 1 out]
        n213 = case shown="No Error" w565 {
          tunnel: w565 -> [w583 w584]
          tunnel: [w582 w584] -> w575
          frame No Error {
            n214 = local read "Output filename"() -> (w578:string)
            n215 = local read "Output path"() -> (w579:path)
            n216 = Path To String(path=w579) -> (string=w581:string)
            n217 = shared-variable "RT CompactRIO Target\\RT_EPICS_Shared_Variables.lvlib\\2iddVELO:VP:Last_Filename"(w578, error in=w583) -> (error out=w580:errorcluster)
            n218 = shared-variable "RT CompactRIO Target\\RT_EPICS_Shared_Variables.lvlib\\2iddVELO:VP:cRIO_Dir"(w581, error in=w580) -> (error out=w582:errorcluster)
          }
          frame Error {
          }
        }
      }
      frame "Restart FPGA" {
        n219 = call <vilib>:"Clear Errors.vi"("error in (no error)"=w590) -> ("error out"=w591:errorcluster)  [unwired: 5 in, 1 out]
        n220 = xnode "Invoke Method"("FPGA VI Reference In"=w596, "error in"=w591) -> ("FPGA VI Reference Out"=w595:refnum<k20>, "error out"=w594:errorcluster)
        n221 = xnode "Read/Write Control"("FPGA VI Reference In"=w595, "error in"=w594, "stop case"=TRUE) -> ("FPGA VI Reference Out"=w589:refnum<k20>, "error out"=w588:errorcluster)
        n222 = xnode "Invoke Method"("FPGA VI Reference In"=w589, "error in"=w588) -> ("FPGA VI Reference Out"=w587:refnum<k20>, "error out"=w586:errorcluster)
      }
      frame "Stop FPGA" {
        w604 = T12[] [enum."Stop FPGA"] items=["Initialization", "Import Controller coeffs", "Update Controller Info", "Wait", "Update Reference Info", "Update Detector Trigger Info", "Update Datalog Info", "Check FPGA Status", "Pre-Scan", "Start Scan", "Scanning", "End Scan", "Restart FPGA", "Stop FPGA"] ("Reduced Array of States")
        w603 = TRUE ("stop case")
        n223 = xnode "Invoke Method"("FPGA VI Reference In"=w611, "error in"=w610) -> ("FPGA VI Reference Out"=w609:refnum<k20>, "error out"=w608:errorcluster)
        n224 = xnode "Read/Write Control"("FPGA VI Reference In"=w609, "error in"=w608, "stop case"=w603, "New FPGA command"=w603, "FPGA command"=enum16{"Start Scan", "Shutdown"}."Shutdown") -> ("FPGA VI Reference Out"=w607:refnum<k20>, "error out"=w600:errorcluster)
        n225 = xnode "Invoke Method"("FPGA VI Reference In"=w607, "error in"=w600) -> ("FPGA VI Reference Out"=w601:refnum<k20>, "error out"=w599:errorcluster)
        n226 = xnode "Close FPGA VI Reference"("FPGA VI Reference In"=w601, "error in"=w599) -> ("error out"=w606:errorcluster)
      }
    }
    "Main Loop error" <- w102
    "Scan loop dt" <- w107
    n227 = shared-variable ".\\Interloop communication.lvlib\\Main Loop Error"(w102) -> ()  [unwired: 1 in, 1 out]
    n228 = node-c288(w107) -> ()  [unwired: 1 out]
    n229 = call "State Control.vi"("Stop"=FALSE, "Array of States"=w112, "Error Input"=w102) -> ("Next State"=w104:T12, "Reduced Array of States"=w108:T12[])  [unwired: 5 in]
    "RT Main Loop State" <- w98
    "Main Loop Iterations" <- w110
    "Reduced Array of States" <- w109
  }
  n230 = while {
    tunnel: w2 -> [w620]
    tunnel: w1 -> [w619]
    i -> [w617]
    stop <- w618 stop-if-true
    # "Readback loop"
    n231 = local read "RT Main Loop State"() -> (w623:T12)
    n232 = Not Equal?(x=w623, y=State_Enum."Initialization") -> (x != y?=w621:bool)
    n233 = case shown="True" w621 {
      tunnel: w620 -> [_ w631]
      tunnel: w619 -> [_ w629]
      tunnel: [u32 100 ("milliseconds to wait") "Readback Loop time between iterations (ms)"] -> w616
      frame False {
      }
      frame True {
        w670 = 40000000.0  # FPGA Clock Rate (Hz)
        w689 = 40000000.0  # FPGA Clock Rate (Hz)
        w706 = 40000000.0  # FPGA Clock Rate (Hz)
        n234 = xnode "Read/Write Control"("FPGA VI Reference In"=w631, "error in"=w629) -> ("FPGA VI Reference Out"=w630:refnum<k20>, "error out"=w628:errorcluster, "FPGA state"=w625:T11, "Fly scan completed"=→"Fly Scan Complete":bool)
        "FPGA state" <- w625
        n235 = Format Into String(format string="%s", w625) -> (resulting string=w627:string)  [unwired: 2 in, 1 out]
        n236 = xnode "Read/Write Control"("FPGA VI Reference In"=w630, "error in"=w628) -> ("error out"=w637:errorcluster, "Measured Datalog Time Period (Ticks)"=w664:u32, "Measured Counter Time Period (Ticks)"=w669:u32, "Mod4/DIO0"=→"Mod4/DIO0":bool, "Mod4/DIO1"=→"Mod4/DIO1":bool, "Mod4/DIO2"=→"Mod4/DIO2":bool, "Mod4/DIO3"=→"Mod4/DIO3":bool, "Mod5/DIO0"=→"Mod5/DIO0":bool, "Mod5/DIO1"=→"Mod5/DIO1":bool, "Mod5/DIO2"=→"Mod5/DIO2":bool, "Mod5/DIO3"=→"Mod5/DIO3":bool, "Mod6/DIO0"=→"Mod6/DIO0":bool, "Mod6/DIO1"=→"Mod6/DIO1":bool, "Mod6/DIO2"=→"Mod6/DIO2":bool, "Mod6/DIO3"=→"Mod6/DIO3":bool, "32 bit Count Optics X"=→"32 bit Count Optics X":i32, "32 bit Count Optics  Y"=→"32 bit Count Optics  Y":i32, "32 bit Count Optics  Z"=→"32 bit Count Optics  Z":i32, "32 bit Count Sample X"=→"32 bit Count Sample X":i32, "32 bit Count Sample  Y"=→"32 bit Count Sample  Y":i32, "32 bit Count Sample  Z"=→"32 bit Count Sample  Z":i32, "Optics X Stage Displacement (nm)"=→"Optics X Stage Displacement (nm)":fxp<+/-,58,25>, "Optics Y Stage Displacement (nm)"=→"Optics Y Stage Displacement (nm)":fxp<+/-,58,25>, "Optics Z Stage Displacement (nm)"=→"Optics Z Stage Displacement (nm)":fxp<+/-,58,25>, "Sample X Stage Displacement (nm)"=→"Sample X Stage Displacement (nm)":fxp<+/-,58,25>, "Sample Y Stage Displacement (nm)"=→"Sample Y Stage Displacement (nm)":fxp<+/-,58,25>, "Sample Z Stage Displacement (nm)"=→"Sample Z Stage Displacement (nm)":fxp<+/-,58,25>)  [unwired: 1 out]
        "Measured Datalog Time Period (Ticks)" <- w664
        "Measured Counter Time Period (Ticks)" <- w669
        n237 = xnode "Read/Write Control"("FPGA VI Reference In"=w630, "error in"=w628) -> ("error out"=w636:errorcluster, "Measured Detector Trigger Time Period (Ticks)"=→"Measured Detector Trigger Time Period (Ticks)":u32, "Measured Trigger Gen Time Period (Ticks)"=→"Measured Trigger Gen Time Period (Ticks)":u32, "Detector Trigger (V)"=→"Detector Trigger (V)":fxp<+/-,20,5>, "Detector Trigger In Range?"=→"Detector Trigger In Range?":bool, "Measured Data Trigger Time Period (Ticks)"=→"Measured Data Trigger Time Period (Ticks)":u32, "Trigger for Data"=→"Trigger for Data":fxp<+/-,58,25>)  [unwired: 1 out]
        n238 = xnode "Read/Write Control"("FPGA VI Reference In"=w630, "error in"=w628) -> ("error out"=w634:errorcluster, "PI X-Stage Input (V)"=→"PI X-Stage Input (V)":fxp<+/-,20,5>, "PI Y-Stage Input (V)"=→"PI Y-Stage Input (V)":fxp<+/-,20,5>, "PI Z-Stage Input (V)"=→"PI Z-Stage Input (V)":fxp<+/-,20,5>, "X-Stage Input In Range?"=→"X-Stage Input In Range?":bool, "Y-Stage Input In Range?"=→"Y-Stage Input In Range?":bool, "Z-Stage Input In Range?"=→"Z-Stage Input In Range?":bool, "Measured Controller Time Period (Ticks)"=w710:u32, "Measured Controller Output Time Period (Ticks)"=w709:u32, "Measured Plant Output Time Period (Ticks)"=w708:u32, "Measured Analog Input Time Period (Ticks)"=w707:u32)  [unwired: 1 out]
        "Measured Controller Time Period (Ticks)" <- w710
        "Measured Controller Output Time Period (Ticks)" <- w709
        "Measured Plant Output Time Period (Ticks)" <- w708
        "Measured Analog Input Time Period (Ticks)" <- w707
        n239 = xnode "Read/Write Control"("FPGA VI Reference In"=w630, "error in"=w628) -> ("error out"=w635:errorcluster, "X Stage Reference (nm)"=→"X Stage Reference (nm)":fxp<+/-,58,25>, "Y Stage Reference (nm)"=→"Y Stage Reference (nm)":fxp<+/-,58,25>, "Z Stage Reference (nm)"=→"Z Stage Reference (nm)":fxp<+/-,58,25>, "Measured X Reference Time Period (Ticks)"=w691:u32, "Measured Y Reference Time Period (Ticks)"=w690:u32, "Measured Z Reference Time Period (Ticks)"=w682:u32, "Fly Scan Running"=→"Fly Scan Running":bool, "Continue Run"=→"Continue Run":bool)  [unwired: 1 out]
        "Measured X Reference Time Period (Ticks)" <- w691
        "Measured Y Reference Time Period (Ticks)" <- w690
        "Measured Z Reference Time Period (Ticks)" <- w682
        n240 = shared-variable "RT CompactRIO Target\\RT_EPICS_Shared_Variables.lvlib\\2iddVELO:VP:FPGA_State"(w627) -> ()  [unwired: 1 in, 1 out]
        n241 = call "Convert Measured Rate.vi"("FPGA Clock Rate (Hz)"=w689, "Measured Reference Time Period (Ticks)"=w682) -> ("Measured Reference Loop Rate (kHz)"=→"Measured Z Reference Loop Rate (kHz)":dbl, "Measured Reference Loop Period (s)"=→"Measured Z Reference Loop Rate (secs)":dbl)
        n242 = call "Convert Measured Rate.vi"("FPGA Clock Rate (Hz)"=w689, "Measured Reference Time Period (Ticks)"=w690) -> ("Measured Reference Loop Rate (kHz)"=→"Measured Y Reference Loop Rate (kHz)":dbl, "Measured Reference Loop Period (s)"=→"Measured Y Reference Loop Rate (secs)":dbl)
        n243 = call "Convert Measured Rate.vi"("FPGA Clock Rate (Hz)"=w670, "Measured Reference Time Period (Ticks)"=w669) -> ("Measured Reference Loop Rate (kHz)"=w667:dbl, "Measured Reference Loop Period (s)"=→"Measured Counter Loop Rate (secs)":dbl)
        n244 = call "Convert Measured Rate.vi"("FPGA Clock Rate (Hz)"=w689, "Measured Reference Time Period (Ticks)"=w691) -> ("Measured Reference Loop Rate (kHz)"=→"Measured X Reference Loop Rate (kHz)":dbl, "Measured Reference Loop Period (s)"=→"Measured X Reference Loop Rate (secs)":dbl)
        n245 = call "Convert Measured Rate.vi"("FPGA Clock Rate (Hz)"=w670, "Measured Reference Time Period (Ticks)"=w664) -> ("Measured Reference Loop Rate (kHz)"=→"Measured Datalog Loop Rate (kHz)":dbl, "Measured Reference Loop Period (s)"=→"Measured Datalog Loop Rate (secs)":dbl)
        n246 = call "Convert Measured Rate.vi"("FPGA Clock Rate (Hz)"=w706, "Measured Reference Time Period (Ticks)"=w710) -> ("Measured Reference Loop Rate (kHz)"=→"Measured Controller Loop Rate (kHz)":dbl, "Measured Reference Loop Period (s)"=→"Measured Controller Loop Rate (secs)":dbl)
        n247 = call "Convert Measured Rate.vi"("FPGA Clock Rate (Hz)"=w706, "Measured Reference Time Period (Ticks)"=w709) -> ("Measured Reference Loop Rate (kHz)"=→"Measured Controller Output Loop Rate (kHz)":dbl, "Measured Reference Loop Period (s)"=→"Measured Controller Output Loop Rate (secs)":dbl)
        n248 = call "Convert Measured Rate.vi"("FPGA Clock Rate (Hz)"=w706, "Measured Reference Time Period (Ticks)"=w708) -> ("Measured Reference Loop Rate (kHz)"=→"Measured Plant Output Loop Rate (kHz)":dbl, "Measured Reference Loop Period (s)"=→"Measured Plant Output Loop Rate (secs)":dbl)
        n249 = call "Convert Measured Rate.vi"("FPGA Clock Rate (Hz)"=w706, "Measured Reference Time Period (Ticks)"=w707) -> ("Measured Reference Loop Rate (kHz)"=→"Measured Analog Input Loop Rate (kHz)":dbl, "Measured Reference Loop Period (s)"=→"Measured Analog Input Loop Rate (secs)":dbl)
        n250 = Divide(x=w667, y=1000.0) -> (x/y=→"Measured Counter Loop Rate (MHz)":dbl)
        n251 = Merge Errors(w634, w635, w636, w637) -> (w633:errorcluster)
        "Readback error" <- w633
        n252 = shared-variable ".\\Interloop communication.lvlib\\Readback Loop Error"(w633) -> ()  [unwired: 1 in, 1 out]
      }
    }
    n253 = local read "Stop System (Careful!!)"() -> (w618:bool)
    n254 = Wait (ms)(milliseconds to wait=w616) -> ()  [unwired: 1 out]
    "Readback loop Iterations" <- w617
  }
  n255 = while {
    stop <- w728 stop-if-true
    n256 = shared-variable "RT CompactRIO Target\\RT_EPICS_Shared_Variables.lvlib\\2iddVELO:VP:Controller_Type"() -> (w726:string, error out=w717:errorcluster)  [unwired: 1 in]
    "2iddVELO:VP:Controller_Type" <- w726
    n257 = shared-variable "RT CompactRIO Target\\RT_EPICS_Shared_Variables.lvlib\\2iddVELO:VP:cRIO_Command"() -> (w725:string, error out=w719:errorcluster)  [unwired: 1 in]
    "2iddVELO:VP:cRIO_Command" <- w725
    n258 = shared-variable "RT CompactRIO Target\\RT_EPICS_Shared_Variables.lvlib\\2iddVELO:VP:Scan_Type"() -> (w723:string, error out=w715:errorcluster)  [unwired: 1 in]
    "2iddVELO:VP:Scan_Type" <- w723
    n259 = Scan From String(input string=w725, error in=w719, default 1=EPICS_Command_Control."Start Scan" ("default value 1")) -> (error out=w718:errorcluster, output 1=→"EPICS cRIO Command":T13)  [unwired: 2 in, 2 out]
    n260 = Scan From String(input string=w726, error in=w717, default 1=Controller_Type."H-infinity" ("Controller Type")) -> (error out=w716:errorcluster, output 1=→"EPICS Controller Type":T3)  [unwired: 2 in, 2 out]
    n261 = Scan From String(input string=w723, error in=w715, default 1=Scan_type."Fly" ("Scan type")) -> (error out=w714:errorcluster, output 1=→"EPICS Scan Type":T2)  [unwired: 2 in, 2 out]
    n262 = local read "Stop System (Careful!!)"() -> (w728:bool)
    n263 = Merge Errors(w718, w716, w714) -> (w713:errorcluster)
    "EPICS command error" <- w713
    n264 = shared-variable ".\\Interloop communication.lvlib\\EPICS command error"(w713) -> ()  [unwired: 1 in, 1 out]
    n265 = Wait Until Next ms Multiple(millisecond multiple=u32 100) -> ()  [unwired: 1 out]
  }
  n266 = node-c288(w8) -> (→"Timed Loop (end error)":errorcluster, →"Iteration Duration RT Timed-Loop":i64)
